vi "MultiSlit_Graphical.vi"() -> (0 "Offsets and Rotation":T7 {"Delta Y" format="%#_4g"; "Delta X" format="%#_4g"; "Delta Theta" format="%#_4g"})   [LabVIEW 2015]
doc: "A graphical tool to provide rotation and offsets needed to align a slit mask with the corresponding field on the sky, using fits images of the mask and field. Based on Brad Barlow's QuickLook software for the Goodman Spectrograph."
uses:
  gfitsio/gfitsio-refnum.ctl
  SystemUtil/Command.ctl
  SIcamera_Globals.vi
  Instance           7 27Saved   MultiSlit_Graphical .vi
  Instance           8 27Saved   MultiSlit_Graphical .vi
panel:
  out "Gauss Fit Window 2":i16[][](array[numeric])
  in  "Zoom Window Width (1/x) 2":u32=10
  out "Display Binning 2":i16
  out "Raw Image Buffer 2":i16[][](array[numeric])
  out "Display Binning":i16
  in  "# of pix to display":i32=200000
  out "Minimum Pix Value":dbl
  out "Maximum Pix Value":dbl
  out "Avg Pix Value":dbl format="%#.1f"
  out "Path to Current File":path
  out "Gauss Fit Window":i16[][](array[numeric])
  in  "Zoom Window Width (1/x)":u32=10
  out "Spectrum Status":string
  out "Image Buffer Info.":T1
  out "error IO":errorcluster
  in  "# of rows at a time":dbl=1.0
  out "Raw Image Buffer 1":i16[][](array[numeric])
  out "Raw Data":T2
  out "gfits refnum":T3
  in  "Tab Control":T4(tab)
  in  "Image Open 2":bool
  out "String 5":string="Center cursor in window - c\nCenter cursor on star or box in zoom window - r\nCenter cursor on slit - a"
  in  "LoadStar":bool
  in  "StarSelection":u16(ring) items=["Star 1", "Star 2", "Star 3"]
  out "String 2":string="Load current coordinates as "
  in  "Autoscale":bool
  in  "Redraw":bool
  in  "Zoom Out":bool
  in  "Zoom In":bool
  out "Y":dbl format="%5.1f"
  out "X":dbl format="%5.1f"
  out "Value":dbl
  out "Zoom Window":i16[][](graph) caption="0051.NGC2808_300line.fits"
  out "Status 1":string
  in  "Image Scale Stretch":cluster{dbl, dbl}(slide)={41.0, 61.0} scale=0.0..100.0
  in  "Image1":dbl[][](graph)=[[0.0]] caption="0008_Fe_ZZCeti_930_blue_long.fits"
  out "String 4":string="Center cursor in window - c\nCenter cursor on star or box in zoom window - r\nCenter cursor on slit - a"
  in  "Image Open":bool
  in  "Image Scale Stretch 2":cluster{dbl, dbl}(slide)={41.0, 61.0} scale=0.0..100.0
  in  "LoadSlit":bool
  in  "SlitSelection":u16(ring) items=["Slit 1", "Slit 2", "Slit 3"]
  out "Test":string="Load current coordinates as "
  in  "Autoscale 2":bool
  in  "Redraw 2":bool
  in  "Zoom Out 2":bool
  in  "Zoom In 2":bool
  out "Y 2":dbl format="%5.1f"
  out "X 2":dbl format="%5.1f"
  out "Value 2":dbl
  out "Zoom Window 2":i16[][](graph) caption="0051.NGC2808_300line.fits"
  out "Status 2":string
  in  "Image2":dbl[][](graph) caption="0267.WASP17b_2100_NaD.fits"
  in  "Set Values to Zero":bool
  out "new y1":dbl
  out "new x1":dbl
  out "String 3":string
  in  "Slit Positions":T5
  in  "Star Positions":T6
  in  "Send Target Offset Position":bool
  in  "Calculate Shifts":bool
  out "FITS Header 2":string
  out "FITS Header":string
  in  "CommandQ":string="MULTISLIT_Q"
  # "X Position"
  # "Y Position"
  # "Star 1"
  # "Star 2"
  # "Star 3"
  # "Slit 1"
  # "Slit 2"
  # "Slit 3"
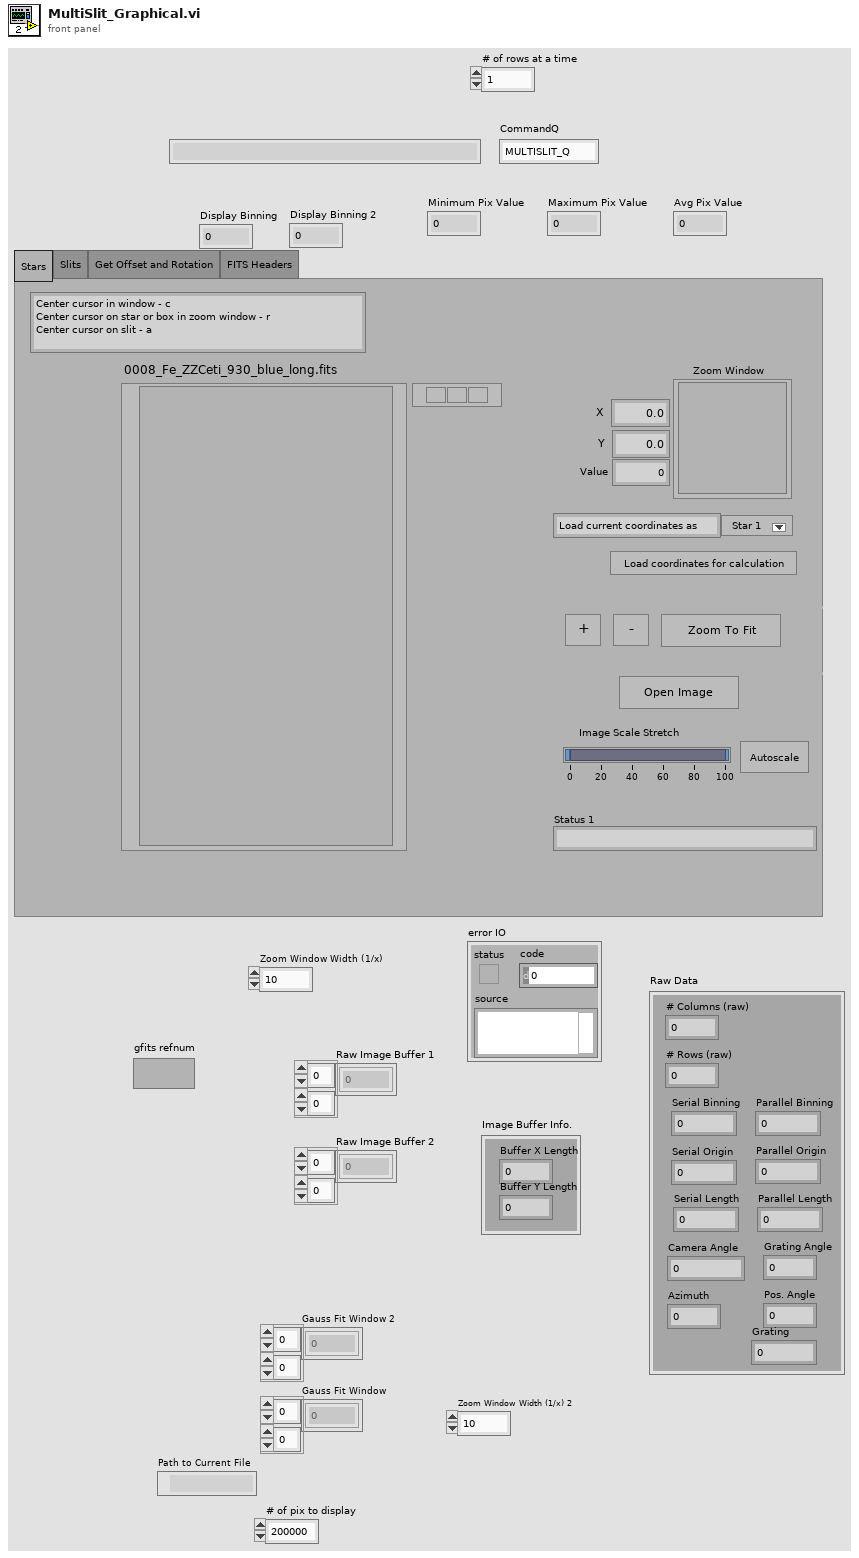
[diagram p1: front panel]
types:
  T1 = cluster{"Buffer X Length":dbl, "Buffer Y Length ":dbl}
  T2 = cluster{"# Columns (raw) ":dbl, "# Rows (raw)":dbl, "Serial Origin":dbl, "Parallel Origin":dbl, "Camera Angle":dbl, "Grating Angle":dbl, "Serial Binning":dbl, "Parallel Binning":dbl, "Azimuth":dbl, "Serial Length":dbl, "Parallel Length":dbl, "Pos. Angle":dbl, "Grating":dbl}
  T3 = typedef "gfitsio-refnum.ctl" = refnum<k1>
  T4 = enum32{"Stars", "Slits", "Get Offset and Rotation", "FITS Headers"}
  T5 = cluster{"Slit x1":dbl, "Slit x2":dbl, "Slit x3":dbl, "Slit y2":dbl, "Slit y3":dbl, "Slit y1":dbl}
  T6 = cluster{"Star x1":dbl, "Star x2":dbl, "Star x3":dbl, "Star y2":dbl, "Star y3":dbl, "Star y1":dbl}
  T7 = cluster{"Delta Theta":dbl, "Delta X":dbl, "Delta Y":dbl}
  T8 = typedef "Command.ctl" = cluster{"Command":string, "Parameter":string}
  T9 = enum32{"existing file", "new file", "new or existing file", "existing dir", "new dir", "new or existing dir", "existing file (use LLBs)", "new file (use LLBs)", "new or existing file (use LLBs)", "new or existing file or directory (use LLBs)"}
  T10 = typedef "LVRangeTypeDef.ctl" = cluster{"Minimum":dbl, "Maximum":dbl, "Increment":dbl, "Minor Increment":dbl, "Start":dbl}
  T11 = typedef "LVPoint32TypeDef.ctl" = cluster{"Horizontal":i32, "Vertical":i32}
  T12 = cluster{"Delta Theta":dbl, "Delta X":dbl, "Delta Y":dbl, "Delta Theta":dbl, "Delta X":dbl, "Delta Y":dbl}
  T13 = typedef "LVPointDoubleTypeDef.ctl" = cluster{"Cursor X":dbl, "Cursor Y":dbl}
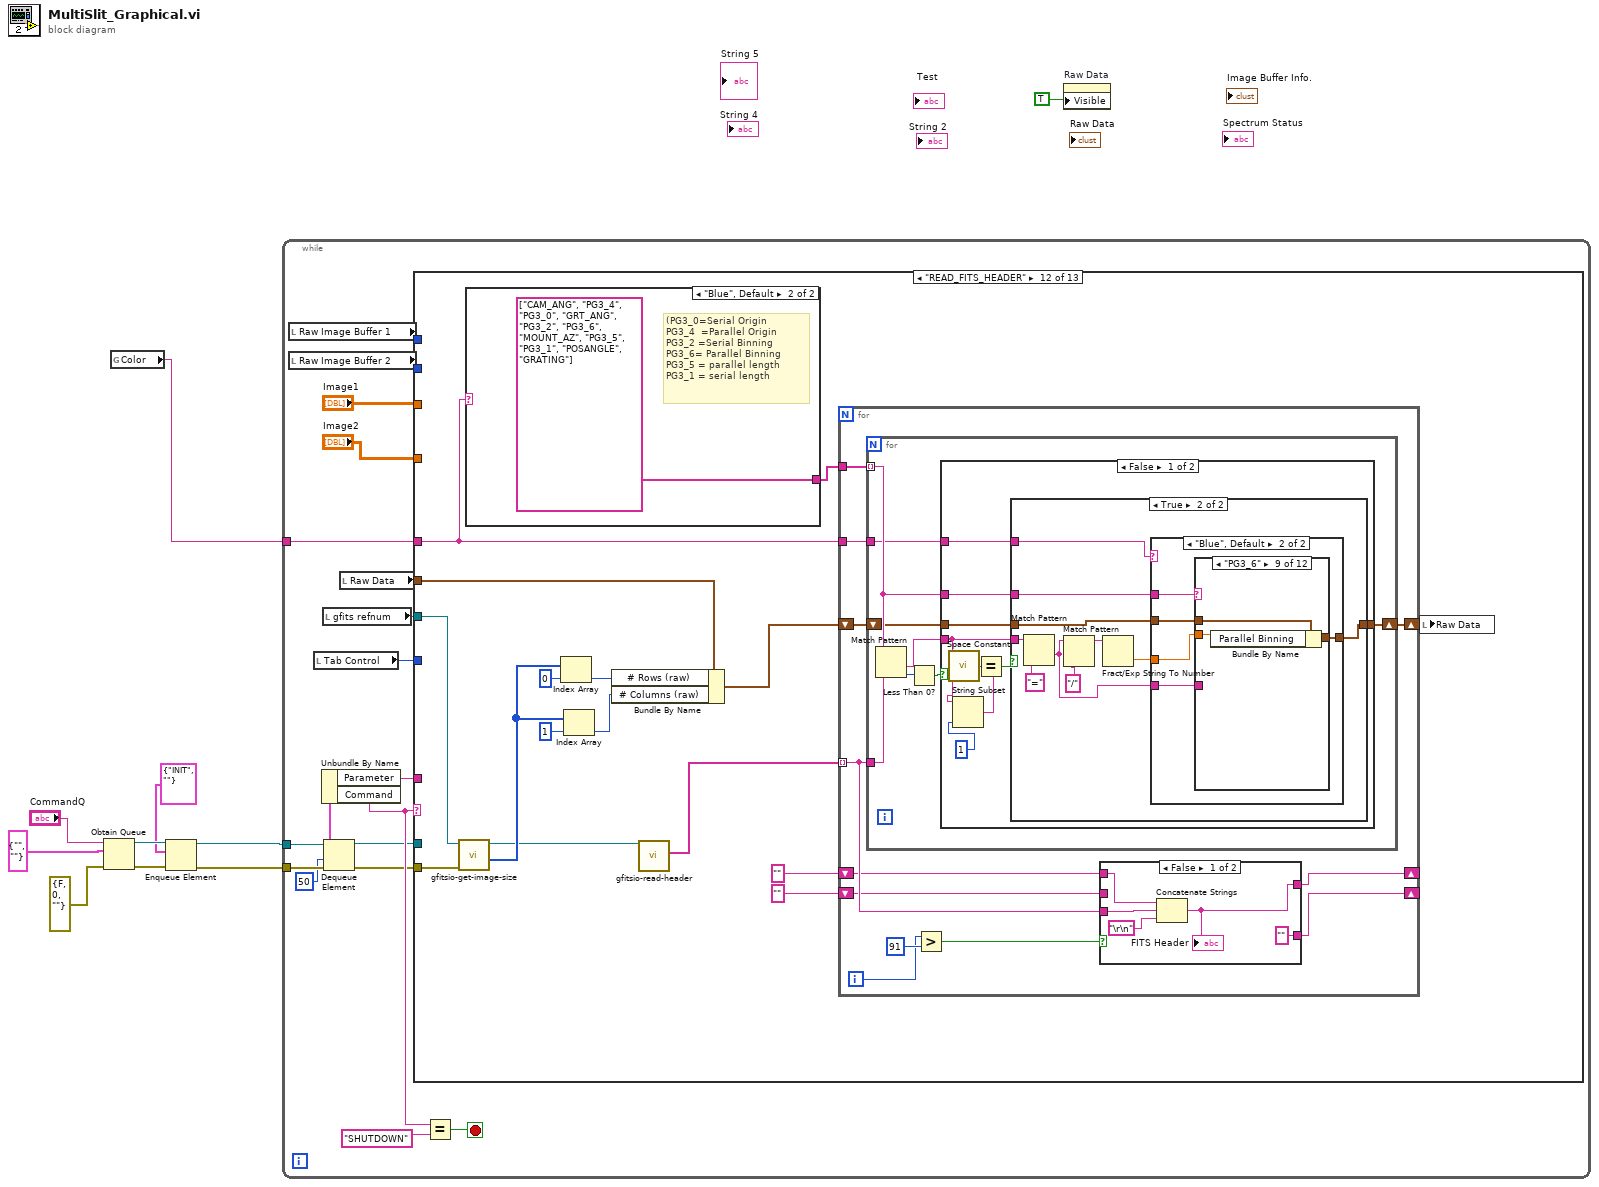
[diagram p0: block diagram]
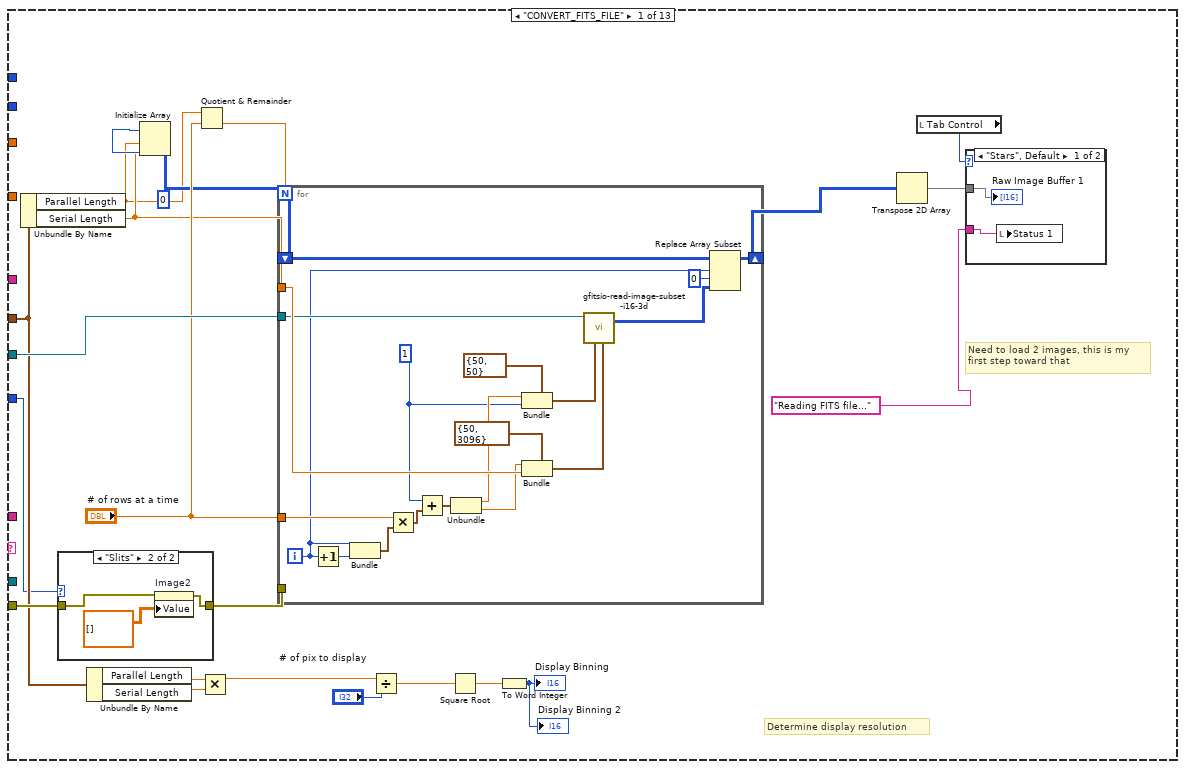
[diagram p2: hidden frame]
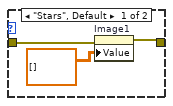
[diagram p3: hidden frame]
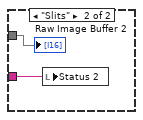
[diagram p4: hidden frame]
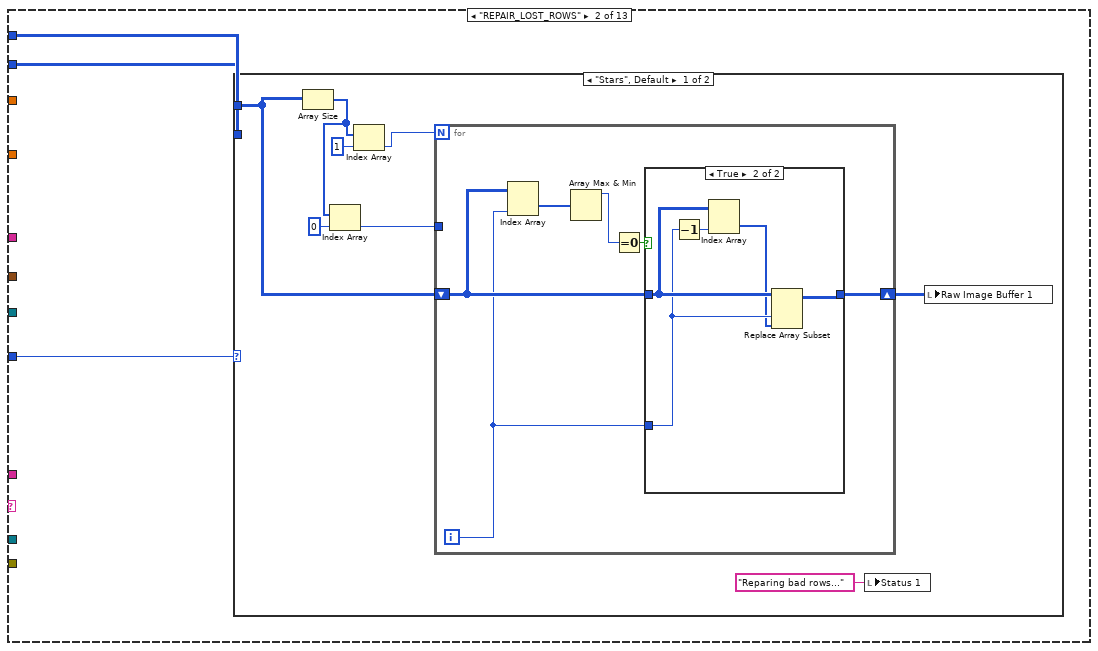
[diagram p5: hidden frame]
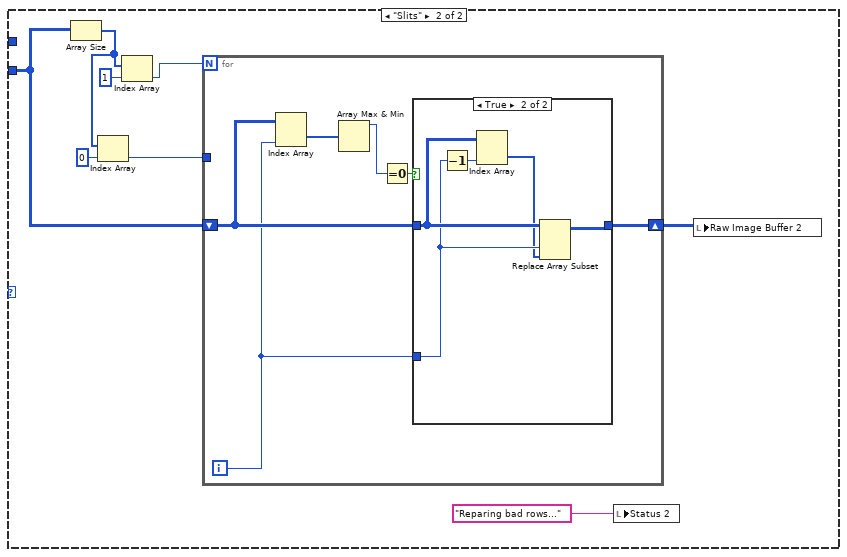
[diagram p7: hidden frame]
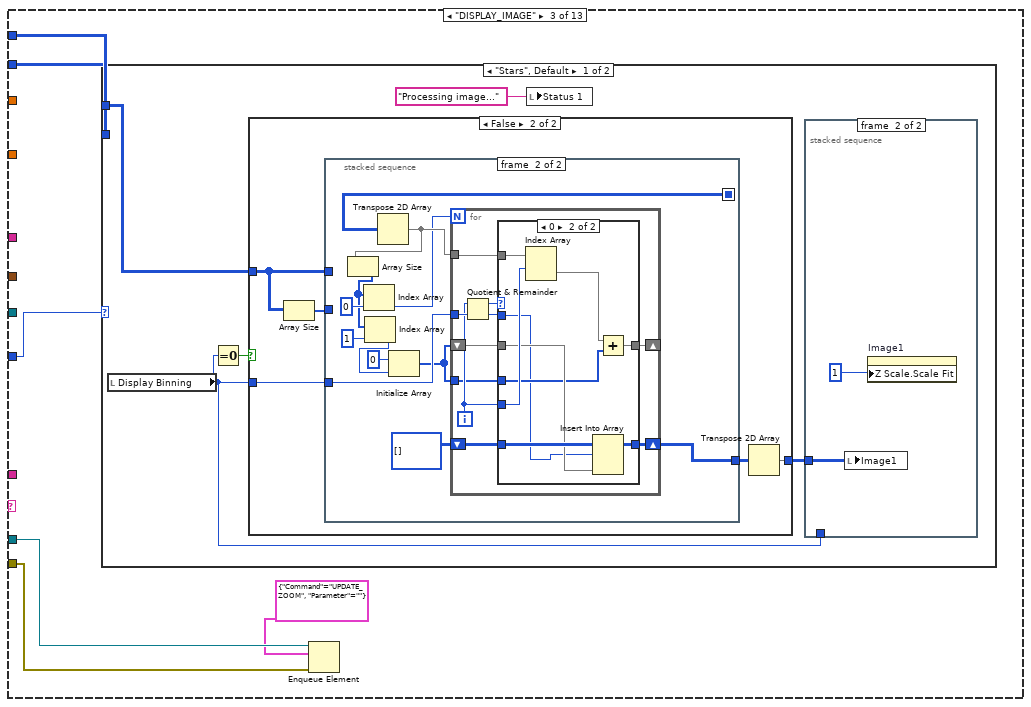
[diagram p9: hidden frame]
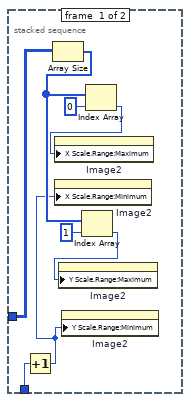
[diagram p10: hidden frame]
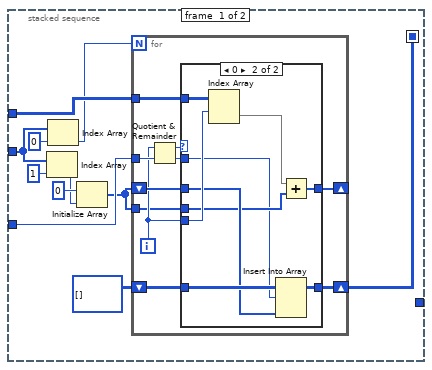
[diagram p12: hidden frame]
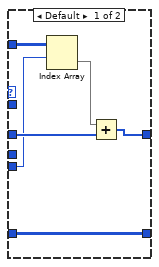
[diagram p13: hidden frame]
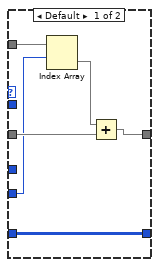
[diagram p14: hidden frame]
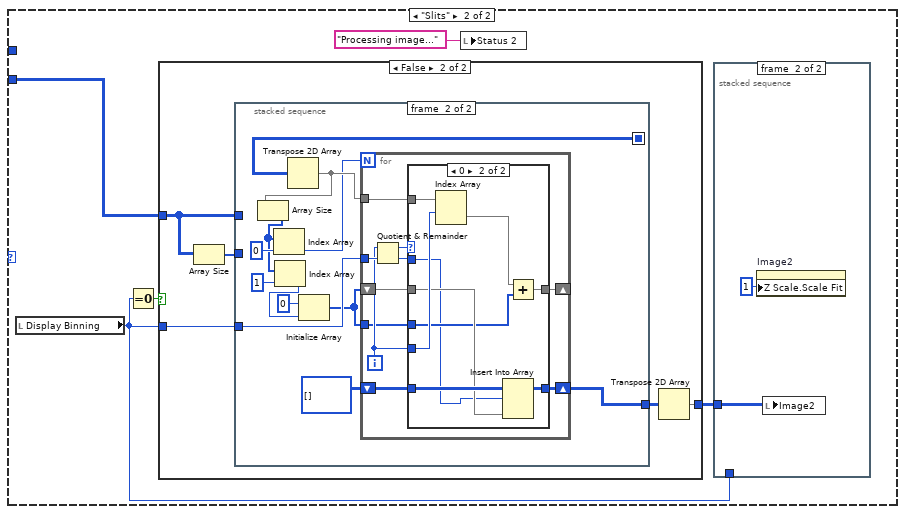
[diagram p15: hidden frame]
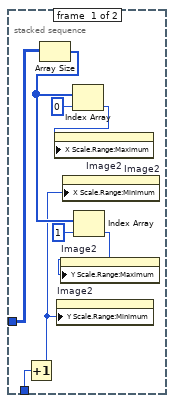
[diagram p16: hidden frame]
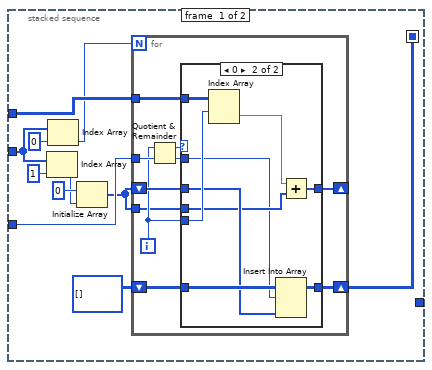
[diagram p18: hidden frame]
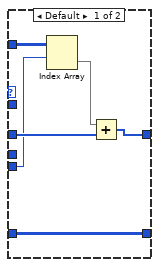
[diagram p19: hidden frame]
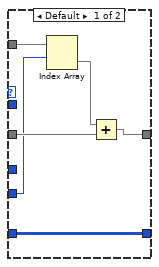
[diagram p20: hidden frame]
diagram:
  n1 = Obtain Queue(name (unnamed)="CommandQ", element data type=T8 {"Command"="", "Parameter"=""} ("Command"), error in (no error)=errorcluster {"status"=FALSE, "code"=0, "source"=""}) -> (queue out=w8:refnum<queue>, error out=w7:errorcluster)  [unwired: 2 in, 1 out]
  n2 = global read "SIcamera_Globals.vi" "Color"() -> (w1:string)
  n3 = Enqueue Element(queue=w8, element=T8 {"Command"="INIT", "Parameter"=""}, error in (no error)=w7) -> (queue out=w5:refnum<queue>, error out=w4:errorcluster)  [unwired: 1 in, 1 out]
  n4 = while {
    tunnel: w4 -> [w28]
    tunnel: w5 -> [w27]
    tunnel: w1 -> [w11]
    stop <- w24 stop-if-true
    n5 = local read "Raw Image Buffer 1"() -> (w15:i16[][])
    n6 = local read "Raw Image Buffer 2"() -> (w14:i16[][])
    n7 = local read "Tab Control"() -> (w13:T4)
    n8 = local read "gfits refnum"() -> (w18:T3)
    n9 = Dequeue Element(queue=w27, timeout in ms (-1)=50, error in (no error)=w28) -> (queue out=w21:refnum<queue>, element=w26:T8, error out=w22:errorcluster)  [unwired: 1 out]
    n10 = Unbundle By Name(w26) -> ("Parameter"=w19:string, "Command"=w23:string)
    n11 = local read "Raw Data"() -> (w17:T2)
    n12 = case shown="\"READ_FITS_HEADER\"" w23 {
      tunnel: w22 -> [w45 _ w125 _ w325 w1011 w1017 _ _ _ w1282 w1325 _]
      tunnel: w21 -> [_ _ w127 _ w326 w1012 w1018 _ _ _ w1281 _ _]
      tunnel: w19 -> [_ _ _ _ _ _ _ _ _ _ w1274 _ _]
      tunnel: "Image1" -> [_ _ _ _ w324 _ _ _ _ _ _ _ _]
      tunnel: w18 -> [w50 _ _ _ _ _ _ _ _ _ _ w1326 _]
      tunnel: w17 -> [w41 _ _ _ w323 _ w1016 _ _ _ _ w1323 _]
      tunnel: w15 -> [_ w82 w128 _ w322 _ _ _ w1147 w1212 _ _ w1474]
      tunnel: w14 -> [_ w81 w123 _ w319 _ _ _ w1146 w1211 _ _ w1473]
      tunnel: w13 -> [w31 w80 w124 _ w320 _ w1013 w1113 w1148 w1213 w1271 _ w1475]
      tunnel: "Image2" -> [_ _ _ _ w321 _ _ _ _ _ _ _ _]
      tunnel: w11 -> [_ _ _ _ _ _ _ _ _ _ _ w1316 _]
      frame "CONVERT_FITS_FILE" {
        # "Need to load 2 images, this is my\nfirst step toward that"
        # "Determine display resolution"
        n13 = Unbundle By Name(w41) -> ("Parallel Length"=w34:dbl, "Serial Length"=w42:dbl)
        n14 = case shown="\"Slits\"" w31 {
          tunnel: [w53 w56] -> w46
          tunnel: w45 -> [w52 w55]
          frame "Stars", Default {
            n15 = property on="Image1" class="IntGraph (strict)"(error in=w52, "Value"=dbl[][] [] ("Image")) -> (error out=w53:errorcluster)  [unwired: 1 in, 1 out]
          }
          frame "Slits" {
            n16 = property on="Image2" class="IntGraph (strict)"(error in=w55, "Value"=dbl[][] [] ("Image")) -> (error out=w56:errorcluster)  [unwired: 1 in, 1 out]
          }
        }
        n17 = Unbundle By Name(w41) -> ("Parallel Length"=w40:dbl, "Serial Length"=w39:dbl)
        n18 = Initialize Array(i16 0 ("element"), w34, w42) -> (w44:i16[][])
        n19 = Quotient & Remainder(x=w34, y="# of rows at a time") -> (floor(x/y)=w49:dbl)  [unwired: 1 out]
        n20 = Multiply(x=w40, y=w39) -> (x*y=w37:dbl)
        n21 = for {
          N: w49 -> [_]
          tunnel: w42 -> [w78]
          tunnel: w50 -> [w68]
          tunnel: "# of rows at a time" -> [w77]
          shift-right: [w65] -> w47
          shift-left: w44 -> [w64]
          tunnel: w46 -> [_]
          i -> [w63]
          w70 = 1
          n22 = Increment(x=w63) -> (x+1=w74:i32)
          n23 = Bundle(w63, w74) -> (w75:cluster{i32, i32})  [unwired: 1 in]
          n24 = Multiply(x=w77, y=w75) -> (x*y=w76:cluster{dbl, dbl})
          n25 = Add(x=w70, y=w76) -> (x+y=w73:cluster{dbl, dbl})
          n26 = Unbundle(w73) -> (w71:dbl, w72:dbl)
          n27 = Bundle(cluster=cluster{i32, i32} {50, 50} ("fpixel (1,1,1)"), w71, w70) -> (w67:cluster{i32, i32})
          n28 = Bundle(cluster=cluster{i32, i32} {50, 3096} ("lpixel (-1,-1,-1: rest)"), w72, w78) -> (w66:cluster{i32, i32})
          n29 = call "gfitsio-read-image-subset-i16-3d.vi"("lpixel (-1,-1,-1: rest)"=w66, "fpixel (1,1,1)"=w67, "gfits refnum"=w68) -> ("data"=w61:i16[][])  [unwired: 5 in, 3 out]
          n30 = Replace Array Subset(array=w64, new element=w61, index (row)=w63, index (col)=0 ("disabled index (col)")) -> (w65:i16[][])
        }
        n31 = Divide(x=w37, y="# of pix to display") -> (x/y=w36:dbl)
        n32 = Square Root(x=w36) -> (sqrt(x)=w35:dbl)
        n33 = To Word Integer(number=w35) -> (16bit integer=→"Display Binning" →"Display Binning 2":i16)
        n34 = Transpose 2D Array(2D array=w47) -> (transposed array=w32:i16[][])
        n35 = local read "Tab Control"() -> (w33:T4)
        n36 = case shown="\"Stars\", Default" w33 {
          tunnel: w32 -> [w58 w60]
          tunnel: "Reading FITS file..." ("Status") -> [w57 w59]
          frame "Stars", Default {
            n37 = local write "Status 1"(w57) -> ()
            "Raw Image Buffer 1" <- w58
          }
          frame "Slits" {
            n38 = local write "Status 2"(w59) -> ()
            "Raw Image Buffer 2" <- w60
          }
        }
      }
      frame "REPAIR_LOST_ROWS" {
        n39 = case shown="\"Stars\", Default" w80 {
          tunnel: w82 -> [w85 _]
          tunnel: w81 -> [_ w105]
          frame "Stars", Default {
            n40 = Array Size(array=w85) -> (size(s)=w87:i32[])
            n41 = Index Array(array=w87, index=0) -> (element=w86:i32)
            n42 = Index Array(array=w87, index=1) -> (element=w89:i32)
            n43 = for {
              N: w89 -> [_]
              shift-right: [w96] -> w84
              shift-left: w85 -> [w95]
              tunnel: w86 -> [_]
              i -> [w94]
              n44 = Index Array(array=w95, index (col)=w94) -> (element=w93:i16[])  [unwired: 1 in]
              n45 = Array Max & Min(array=w93) -> (max value=w91:i16)  [unwired: 3 out]
              n46 = Equal To 0?(x=w91) -> (x = 0?=w92:bool)
              n47 = case shown="True" w92 {
                tunnel: w94 -> [_ w99]
                tunnel: w95 -> [w97 w101]
                tunnel: [w97 w102] -> w96
                frame False {
                }
                frame True {
                  n48 = Decrement(x=w99) -> (x-1=w100:i32)
                  n49 = Index Array(array=w101, index (col)=w100) -> (element=w98:i16[])  [unwired: 1 in]
                  n50 = Replace Array Subset(array=w101, new element=w98, index (col)=w99) -> (w102:i16[][])  [unwired: 1 in]
                }
              }
            }
            n51 = local write "Status 1"("Reparing bad rows..." ("Image Status")) -> ()
            n52 = local write "Raw Image Buffer 1"(w84) -> ()
          }
          frame "Slits" {
            n53 = Array Size(array=w105) -> (size(s)=w107:i32[])
            n54 = Index Array(array=w107, index=0) -> (element=w106:i32)
            n55 = Index Array(array=w107, index=1) -> (element=w109:i32)
            n56 = for {
              N: w109 -> [_]
              shift-right: [w116] -> w104
              shift-left: w105 -> [w115]
              tunnel: w106 -> [_]
              i -> [w114]
              n57 = Index Array(array=w115, index (col)=w114) -> (element=w113:i16[])  [unwired: 1 in]
              n58 = Array Max & Min(array=w113) -> (max value=w111:i16)  [unwired: 3 out]
              n59 = Equal To 0?(x=w111) -> (x = 0?=w112:bool)
              n60 = case shown="True" w112 {
                tunnel: w114 -> [_ w119]
                tunnel: w115 -> [w117 w121]
                tunnel: [w117 w122] -> w116
                frame False {
                }
                frame True {
                  n61 = Decrement(x=w119) -> (x-1=w120:i32)
                  n62 = Index Array(array=w121, index (col)=w120) -> (element=w118:i16[])  [unwired: 1 in]
                  n63 = Replace Array Subset(array=w121, new element=w118, index (col)=w119) -> (w122:i16[][])  [unwired: 1 in]
                }
              }
            }
            n64 = local write "Status 2"("Reparing bad rows..." ("Image Status")) -> ()
            n65 = local write "Raw Image Buffer 2"(w104) -> ()
          }
        }
      }
      frame "DISPLAY_IMAGE" {
        n66 = case shown="\"Stars\", Default" w124 {
          tunnel: w128 -> [w132 _]
          tunnel: w123 -> [_ w223]
          frame "Stars", Default {
            n67 = local read "Display Binning"() -> (w130:i16)
            n68 = Equal To 0?(x=w130) -> (x = 0?=w131:bool)
            n69 = case shown="False" w131 {
              tunnel: w132 -> [w144 w148]
              tunnel: w130 -> [_ w147]
              tunnel: [w144 w146] -> w129
              frame True {
              }
              frame False {
                n70 = Array Size(array=w148) -> (size(s)=w149:i32[])
                n71 = stacked-sequence {
                  seq-local: [w158 _] -> [_ w195]
                  tunnel: w148 -> [w160 _]
                  tunnel: w149 -> [w152 _]
                  tunnel: w147 -> [w156 w192]
                  tunnel: [_ w196] -> w145
                  frame #0 {
                    n72 = Index Array(array=w152, index=1) -> (element=w151:i32)
                    n73 = Index Array(array=w152, index=0) -> (element=w154:i32)
                    n74 = Initialize Array(0 ("element"), w151) -> (w150:i32[])
                    n75 = for {
                      N: w154 -> [_]
                      tunnel: w160 -> [w170]
                      shift-right: [w168] -> w158
                      shift-left: i32[][] [] -> [w169]
                      tunnel: w156 -> [w167]
                      shift-right: [w163] -> _
                      shift-left: w150 -> [w164]
                      tunnel: w150 -> [w161]
                      i -> [w162]
                      n76 = Quotient & Remainder(x=w162, y=w167) -> (x-y*floor(x/y)=w166:i32, floor(x/y)=w165:i32)
                      n77 = case shown="0" w166 {
                        tunnel: w170 -> [w176 w185]
                        tunnel: w162 -> [w172 w182]
                        tunnel: w169 -> [w171 w184]
                        tunnel: [w171 w183] -> w168
                        tunnel: w165 -> [_ w177]
                        tunnel: w164 -> [w174 w181]
                        tunnel: [w173 w179] -> w163
                        tunnel: w161 -> [_ w178]
                        frame Default {
                          n78 = Index Array(array=w176, index (row)=w172) -> (element=w175:i16[])  [unwired: 1 in]
                          n79 = Add(x=w175, y=w174) -> (x+y=w173:i32[])
                        }
                        frame 0 {
                          n80 = Index Array(array=w185, index (row)=w182) -> (element=w180:i16[])  [unwired: 1 in]
                          n81 = Insert Into Array(array=w184, index (row)=w177, new element=w181) -> (w183:i32[][])  [unwired: 1 in]
                          n82 = Add(x=w180, y=w178) -> (x+y=w179:i32[])
                        }
                      }
                    }
                  }
                  frame #1 {
                    n83 = Transpose 2D Array(2D array=w195) -> (transposed array=w193:i32[][])
                    n84 = Array Size(array=w193) -> (size(s)=w187:i32[])
                    n85 = Index Array(array=w187, index=0) -> (element=w190:i32)
                    n86 = Index Array(array=w187, index=1) -> (element=w188:i32)
                    n87 = Initialize Array(0 ("element"), w188) -> (w186:i32[])
                    n88 = for {
                      N: w190 -> [_]
                      tunnel: w193 -> [w207]
                      shift-right: [w200] -> w196
                      shift-left: i32[][] [] -> [w201]
                      shift-right: [w206] -> _
                      shift-left: w186 -> [w205]
                      tunnel: w192 -> [w202]
                      tunnel: w186 -> [w198]
                      i -> [w199]
                      n89 = Quotient & Remainder(x=w199, y=w202) -> (x-y*floor(x/y)=w204:i32, floor(x/y)=w203:i32)
                      n90 = case shown="0" w204 {
                        tunnel: w207 -> [w213 w222]
                        tunnel: w199 -> [w209 w219]
                        tunnel: w201 -> [w208 w221]
                        tunnel: [w208 w220] -> w200
                        tunnel: w203 -> [_ w214]
                        tunnel: w205 -> [w211 w218]
                        tunnel: [w210 w216] -> w206
                        tunnel: w198 -> [_ w215]
                        frame Default {
                          n91 = Index Array(array=w213, index (row)=w209) -> (element=w212:i32[])  [unwired: 1 in]
                          n92 = Add(x=w212, y=w211) -> (x+y=w210:i32[])
                        }
                        frame 0 {
                          n93 = Index Array(array=w222, index (row)=w219) -> (element=w217:i32[])  [unwired: 1 in]
                          n94 = Insert Into Array(array=w221, index (row)=w214, new element=w218) -> (w220:i32[][])  [unwired: 1 in]
                          n95 = Add(x=w217, y=w215) -> (x+y=w216:i32[])
                        }
                      }
                    }
                  }
                }
                n96 = Transpose 2D Array(2D array=w145) -> (transposed array=w146:i32[][])
              }
            }
            n97 = local write "Status 1"("Processing image..." ("Status")) -> ()
            n98 = stacked-sequence {
              tunnel: w130 -> [w139 _]
              tunnel: w129 -> [w140 w143]
              frame #0 {
                n99 = Increment(x=w139) -> (x+1=w134:i16)
                n100 = Array Size(array=w140) -> (size(s)=w136:i32[])
                n101 = property on="Image2" class="IntGraph (strict)"("X Scale.Range:Minimum"=w134) -> ()  [unwired: 2 in, 2 out]
                n102 = property on="Image2" class="IntGraph (strict)"("Y Scale.Range:Minimum"=w134) -> ()  [unwired: 2 in, 2 out]
                n103 = Index Array(array=w136, index=1) -> (element=w135:i32)
                n104 = property on="Image2" class="IntGraph (strict)"("Y Scale.Range:Maximum"=w135) -> ()  [unwired: 2 in, 2 out]
                n105 = Index Array(array=w136, index=0) -> (element=w138:i32)
                n106 = property on="Image2" class="IntGraph (strict)"("X Scale.Range:Maximum"=w138) -> ()  [unwired: 2 in, 2 out]
              }
              frame #1 {
                n107 = local write "Image1"(w143) -> ()
                n108 = property on="Image1" class="IntGraph (strict)"("Z Scale.Scale Fit"=1) -> ()  [unwired: 2 in, 2 out]
              }
            }
          }
          frame "Slits" {
            n109 = local read "Display Binning"() -> (w224:i16)
            n110 = Equal To 0?(x=w224) -> (x = 0?=w226:bool)
            n111 = case shown="False" w226 {
              tunnel: w223 -> [w238 w242]
              tunnel: w224 -> [_ w241]
              tunnel: [w238 w240] -> w225
              frame True {
              }
              frame False {
                n112 = Array Size(array=w242) -> (size(s)=w243:i32[])
                n113 = stacked-sequence {
                  seq-local: [w252 _] -> [_ w289]
                  tunnel: w242 -> [w254 _]
                  tunnel: w243 -> [w246 _]
                  tunnel: w241 -> [w250 w286]
                  tunnel: [_ w290] -> w239
                  frame #0 {
                    n114 = Index Array(array=w246, index=1) -> (element=w245:i32)
                    n115 = Index Array(array=w246, index=0) -> (element=w248:i32)
                    n116 = Initialize Array(0 ("element"), w245) -> (w244:i32[])
                    n117 = for {
                      N: w248 -> [_]
                      tunnel: w254 -> [w264]
                      shift-right: [w262] -> w252
                      shift-left: i32[][] [] -> [w263]
                      tunnel: w250 -> [w261]
                      shift-right: [w257] -> _
                      shift-left: w244 -> [w258]
                      tunnel: w244 -> [w255]
                      i -> [w256]
                      n118 = Quotient & Remainder(x=w256, y=w261) -> (x-y*floor(x/y)=w260:i32, floor(x/y)=w259:i32)
                      n119 = case shown="0" w260 {
                        tunnel: w264 -> [w270 w279]
                        tunnel: w256 -> [w266 w276]
                        tunnel: w263 -> [w265 w278]
                        tunnel: [w265 w277] -> w262
                        tunnel: w259 -> [_ w271]
                        tunnel: w258 -> [w268 w275]
                        tunnel: [w267 w273] -> w257
                        tunnel: w255 -> [_ w272]
                        frame Default {
                          n120 = Index Array(array=w270, index (row)=w266) -> (element=w269:i16[])  [unwired: 1 in]
                          n121 = Add(x=w269, y=w268) -> (x+y=w267:i32[])
                        }
                        frame 0 {
                          n122 = Index Array(array=w279, index (row)=w276) -> (element=w274:i16[])  [unwired: 1 in]
                          n123 = Insert Into Array(array=w278, index (row)=w271, new element=w275) -> (w277:i32[][])  [unwired: 1 in]
                          n124 = Add(x=w274, y=w272) -> (x+y=w273:i32[])
                        }
                      }
                    }
                  }
                  frame #1 {
                    n125 = Transpose 2D Array(2D array=w289) -> (transposed array=w287:i32[][])
                    n126 = Array Size(array=w287) -> (size(s)=w281:i32[])
                    n127 = Index Array(array=w281, index=0) -> (element=w284:i32)
                    n128 = Index Array(array=w281, index=1) -> (element=w282:i32)
                    n129 = Initialize Array(0 ("element"), w282) -> (w280:i32[])
                    n130 = for {
                      N: w284 -> [_]
                      tunnel: w287 -> [w301]
                      shift-right: [w294] -> w290
                      shift-left: i32[][] [] -> [w295]
                      shift-right: [w300] -> _
                      shift-left: w280 -> [w299]
                      tunnel: w286 -> [w296]
                      tunnel: w280 -> [w292]
                      i -> [w293]
                      n131 = Quotient & Remainder(x=w293, y=w296) -> (x-y*floor(x/y)=w298:i32, floor(x/y)=w297:i32)
                      n132 = case shown="0" w298 {
                        tunnel: w301 -> [w307 w316]
                        tunnel: w293 -> [w303 w313]
                        tunnel: w295 -> [w302 w315]
                        tunnel: [w302 w314] -> w294
                        tunnel: w297 -> [_ w308]
                        tunnel: w299 -> [w305 w312]
                        tunnel: [w304 w310] -> w300
                        tunnel: w292 -> [_ w309]
                        frame Default {
                          n133 = Index Array(array=w307, index (row)=w303) -> (element=w306:i32[])  [unwired: 1 in]
                          n134 = Add(x=w306, y=w305) -> (x+y=w304:i32[])
                        }
                        frame 0 {
                          n135 = Index Array(array=w316, index (row)=w313) -> (element=w311:i32[])  [unwired: 1 in]
                          n136 = Insert Into Array(array=w315, index (row)=w308, new element=w312) -> (w314:i32[][])  [unwired: 1 in]
                          n137 = Add(x=w311, y=w309) -> (x+y=w310:i32[])
                        }
                      }
                    }
                  }
                }
                n138 = Transpose 2D Array(2D array=w239) -> (transposed array=w240:i32[][])
              }
            }
            n139 = local write "Status 2"("Processing image..." ("Status")) -> ()
            n140 = stacked-sequence {
              tunnel: w225 -> [w230 w237]
              tunnel: w224 -> [w229 _]
              frame #0 {
                n141 = Increment(x=w229) -> (x+1=w228:i16)
                n142 = Array Size(array=w230) -> (size(s)=w233:i32[])
                n143 = property on="Image2" class="IntGraph (strict)"("Y Scale.Range:Minimum"=w228) -> ()  [unwired: 2 in, 2 out]
                n144 = property on="Image2" class="IntGraph (strict)"("X Scale.Range:Minimum"=w228) -> ()  [unwired: 2 in, 2 out]
                n145 = Index Array(array=w233, index=0) -> (element=w234:i32)
                n146 = property on="Image2" class="IntGraph (strict)"("X Scale.Range:Maximum"=w234) -> ()  [unwired: 2 in, 2 out]
                n147 = Index Array(array=w233, index=1) -> (element=w231:i32)
                n148 = property on="Image2" class="IntGraph (strict)"("Y Scale.Range:Maximum"=w231) -> ()  [unwired: 2 in, 2 out]
              }
              frame #1 {
                n149 = property on="Image2" class="IntGraph (strict)"("Z Scale.Scale Fit"=u8 1) -> ()  [unwired: 2 in, 2 out]
                n150 = local write "Image2"(w237) -> ()
              }
            }
          }
        }
        n151 = Enqueue Element(queue=w127, element=T8 {"Command"="UPDATE_ZOOM", "Parameter"=""}, error in (no error)=w125) -> ()  [unwired: 1 in, 3 out]
      }
      frame "INIT" {
        w317 = dbl[][] [[0.0]] ("Image")
        w318 = dbl[][] [[0.0]] ("Image")
        n152 = local write "Zoom Window"(w318) -> ()
        n153 = local write "Image1"(w318) -> ()
        n154 = local write "Zoom Window 2"(w317) -> ()
        n155 = local write "Image2"(w317) -> ()
      }
      frame "", Default {
        n156 = event shown="[2] Menu Selection (User)" {
          selector: _ -> [_ _ _ _ _ _ _ _ _ _ _ _ _ _ _ _ _ _ _ _ _ _ _]
          dyn-events: _ -> [_ _ _ _ _ _ _ _ _ _ _ _ _ _ _ _ _ _ _ _ _ _ _]
          timeout: 50 -> [_ _ _ _ _ _ _ _ _ _ _ _ _ _ _ _ _ _ _ _ _ _ _]
          tunnel: w326 -> [_ w342 w349 _ _ w411 w415 w431 w445 w451 _ _ _ _ _ w884 w914 _ _ w976 w979 _ _]
          tunnel: w325 -> [_ w343 w348 _ _ w412 w414 w430 w444 w452 _ _ _ _ _ w885 w913 _ _ w975 w978 _ _]
          tunnel: w324 -> [_ _ _ _ _ _ _ _ _ w448 _ _ _ _ _ w886 _ _ _ _ _ _ _]
          tunnel: w323 -> [_ _ _ _ _ _ _ _ _ w450 _ _ _ _ _ _ _ _ _ _ _ _ _]
          tunnel: w322 -> [_ w341 _ _ _ _ _ _ _ _ _ _ _ _ _ _ _ _ _ _ _ _ _]
          tunnel: w321 -> [_ _ _ _ _ _ _ _ _ w447 _ _ _ _ _ _ _ _ _ _ _ _ _]
          tunnel: w320 -> [_ _ _ _ _ _ _ _ _ w453 _ _ _ _ _ _ _ _ _ _ _ _ _]
          tunnel: w319 -> [_ w340 _ _ _ _ _ _ _ _ _ _ _ _ _ _ _ _ _ _ _ _ _]
          event Timeout {
            n157 = event-data() -> ()  [unwired: 1 in, 2 out]
            n158 = local read "Status 2"() -> (w329:string)
            n159 = local read "Status 1"() -> (w331:string)
            n160 = case shown="Default" w331 {
              selector: w331 -> [w336 _ _ _]
              tunnel: [w336 "DONE:  Image updated" ("Image Status") "DONE:  Image re-scaled" ("Image Status") "DONE:  Star centered" ("Image Status")] -> w330
              frame Default {
              }
              frame "Processing image..." {
              }
              frame "Scaling image..." {
              }
              frame "Centering star..." {
              }
            }
            "Status 1" <- w330
            n161 = case shown="Default" w329 {
              selector: w329 -> [w332 _ _ _]
              tunnel: [w332 "DONE:  Image updated" ("Image Status") "DONE:  Image re-scaled" ("Image Status") "DONE:  Star centered" ("Image Status")] -> w328
              frame Default {
              }
              frame "Processing image..." {
              }
              frame "Scaling image..." {
              }
              frame "Centering star..." {
              }
            }
            "Status 2" <- w328
          }
          event "Tab Control": Value Change {
            n162 = event-data() -> ("NewVal"=w344:T4)  [unwired: 1 in]
            n163 = case shown="\"Get Offset and Rotation\"" w344 {
              tunnel: w341 -> [_ _ _ _]
              tunnel: w343 -> [_ _ _ w346]
              tunnel: w342 -> [_ _ _ w345]
              tunnel: w340 -> [_ _ _ _]
              frame "Stars", Default {
              }
              frame "Slits" {
              }
              frame "Get Offset and Rotation" {
              }
              frame "FITS Headers" {
                n164 = Enqueue Element(queue=w345, element=T8 {"Command"="GET_IMAGE_STATS", "Parameter"=""}, error in (no error)=w346) -> ()  [unwired: 1 in, 3 out]
              }
            }
          }
          event Menu Selection (User) {
            n165 = event-data() -> ("ItemTag"=w350:string)  [unwired: 1 in]
            n166 = case shown="\"COPY_OTHER\"" w350 {
              tunnel: w349 -> [_ w353 _ _ w393 _ _]
              tunnel: w348 -> [_ w352 _ _ w394 _ _]
              frame "", Default {
              }
              frame "EXIT" {
                n167 = Enqueue Element(queue=w353, element=T8 {"Command"="SHUTDOWN", "Parameter"=""}, error in (no error)=w352) -> ()  [unwired: 1 in, 3 out]
              }
              frame "COPY_CURRENT" {
                w359 = " " ("string")
                n168 = local read "Path to Current File"() -> (w365:path)
                n169 = Strip Path(path=w365) -> (name=w364:string)  [unwired: 1 out]
                n170 = Path To String(path=w365) -> (string=w360:string)
                n171 = Concatenate Strings("\\\\soaric7.ctio.noao.edu\\ic7home3\\observer\\today\\" ("string"), w364) -> (w358:string)
                n172 = Concatenate Strings("cmd /C" ("string"), w359, "copy" ("string"), w359, w360, w359, w358) -> (w357:string)
                n173 = call <vilib>:"System Exec.vi"("run minimized? (F)"=TRUE, "wait until completion? (T)"=TRUE, "command line"=w357) -> ("standard output"=w354:string)  [unwired: 5 in, 3 out]
                n174 = local write "Status 1"(w354) -> ()
              }
              frame "COPY_OTHER" {
                (unwired) T9."existing file" ("select mode (2)")
                n175 = File Dialog(5:"Copy to IC7" ("button label"), 6:"*.fits" ("default name"), 7:"Select an Image to Copy to Soaric7" ("prompt"), 11:path "C:/DATA" ("start path")) -> (0:w366:errorcluster, 1:w368:bool, 3:w369:path)  [unwired: 3 in, 1 out]
                n176 = Unbundle(w366) -> ()  [unwired: 3 out]
                n177 = case shown="False" w368 {
                  tunnel: w369 -> [_ w374]
                  frame True {
                  }
                  frame False {
                    w380 = " " ("string")
                    n178 = Strip Path(path=w374) -> (name=w384:string)  [unwired: 1 out]
                    n179 = Path To String(path=w374) -> (string=w381:string)
                    n180 = Concatenate Strings("\\\\soaric7.ctio.noao.edu\\ic7home3\\observer\\today\\" ("string"), w384) -> (w379:string)
                    n181 = Concatenate Strings("cmd /C" ("string"), w380, "copy" ("string"), w380, w381, w380, w379) -> (w378:string)
                    n182 = call <vilib>:"System Exec.vi"("run minimized? (F)"=TRUE, "wait until completion? (T)"=TRUE, "command line"=w378) -> ("standard output"=w373:string)  [unwired: 5 in, 3 out]
                    n183 = local write "Status 1"(w373) -> ()
                  }
                }
              }
              frame "OPEN" {
                (unwired) T9."existing file" ("select mode (2)")
                n184 = File Dialog(5:"Open Image" ("button label"), 6:"*.fits" ("default name"), 7:"Open Image" ("prompt"), 11:path "C:/DATA" ("start path")) -> (0:w385:errorcluster, 1:w392:bool, 3:w386:path)  [unwired: 3 in, 1 out]
                n185 = Unbundle(w385) -> ()  [unwired: 3 out]
                n186 = Path To String(path=w386) -> (string=w387:string)
                n187 = case shown="False" w392 {
                  tunnel: w394 -> [_ w400]
                  tunnel: w393 -> [_ w399]
                  tunnel: w387 -> [_ w397]
                  frame True {
                  }
                  frame False {
                    n188 = Bundle By Name(cluster=T8 {"Command"="", "Parameter"=""} ("element"), "Command"="OPEN_FITS_FILE", "Parameter"=w397) -> (w398:T8)
                    n189 = Enqueue Element(queue=w399, element=w398, error in (no error)=w400) -> ()  [unwired: 1 in, 3 out]
                  }
                }
              }
              frame "CONFIG" {
                n190 = call "Configuration Parameters"() -> ("# of pixels to display"=w401:dbl, "OK"=w402:bool)  [unwired: 17 in, 1 out]
                n191 = case shown="True" w402 {
                  tunnel: w401 -> [_ w404]
                  frame False {
                  }
                  frame True {
                    w405 = 40000.0 ("y")
                    n192 = Less?(x=w404, y=w405) -> (x < y?=w406:bool)
                    n193 = Select(t=w405, s=w406, f=w404) -> (s? t:f=w403:dbl)
                    n194 = local write "# of pix to display"(w403) -> ()
                  }
                }
              }
              frame "QUICK_HELP" {
                n195 = call "Display Message to User"() -> ()  [unwired: 10 in, 2 out]
              }
            }
          }
          event "Autoscale": Value Change {
            n196 = event-data() -> ()  [unwired: 1 in, 6 out]
            n197 = property on="Image1" class="IntGraph (strict)"("Z Scale.Scale Fit"=u8 1) -> ()  [unwired: 2 in, 2 out]
            n198 = local write "Autoscale"(FALSE ("Autoscale")) -> ()
          }
          event "Autoscale 2": Value Change {
            n199 = event-data() -> ()  [unwired: 1 in, 6 out]
            n200 = property on="Image2" class="IntGraph (strict)"("Z Scale.Scale Fit"=u8 1) -> ()  [unwired: 2 in, 2 out]
            n201 = local write "Autoscale 2"(FALSE ("Autoscale")) -> ()
          }
          event "Redraw": Mouse Down {
            n202 = event-data() -> ()  [unwired: 1 in, 8 out]
            n203 = Enqueue Element(queue=w411, element=T8 {"Command"="DISPLAY_IMAGE", "Parameter"=""}, error in (no error)=w412) -> ()  [unwired: 1 in, 3 out]
          }
          event "Image Open": Mouse Down {
            n204 = event-data() -> ()  [unwired: 1 in, 8 out]
            n205 = case shown="True" "Image Open" {
              tunnel: w414 -> [w421 _]
              tunnel: w415 -> [w420 _]
              frame True {
                (unwired) T9."existing file" ("select mode (2)")
                n206 = File Dialog(5:"Open Image" ("button label"), 6:"*.fits" ("default name"), 7:"Open Image" ("prompt"), 11:path "C:/DATA" ("start path")) -> (0:w417:errorcluster, 3:w423:path)  [unwired: 3 in, 2 out]
                n207 = Unbundle(w417) -> ()  [unwired: 3 out]
                n208 = Path To String(path=w423) -> (string=w422:string)
                n209 = Bundle By Name(cluster=T8 {"Command"="", "Parameter"=""} ("element"), "Command"="OPEN_FITS_FILE", "Parameter"=w422) -> (w419:T8)
                n210 = Enqueue Element(queue=w420, element=w419, error in (no error)=w421) -> ()  [unwired: 1 in, 3 out]
              }
              frame False {
              }
            }
          }
          event "Image Open 2": Mouse Down {
            n211 = event-data() -> ()  [unwired: 1 in, 8 out]
            n212 = case shown="True" "Image Open 2" {
              tunnel: w430 -> [w436 _]
              tunnel: w431 -> [w435 _]
              frame True {
                (unwired) T9."existing file" ("select mode (2)")
                n213 = File Dialog(5:"Open Image" ("button label"), 6:"*.fits" ("default name"), 7:"Open Image" ("prompt"), 11:path "C:/DATA" ("start path")) -> (0:w432:errorcluster, 3:w438:path)  [unwired: 3 in, 2 out]
                n214 = Unbundle(w432) -> ()  [unwired: 3 out]
                n215 = Path To String(path=w438) -> (string=w437:string)
                n216 = Bundle By Name(cluster=T8 {"Command"="", "Parameter"=""} ("element"), "Command"="OPEN_FITS_FILE", "Parameter"=w437) -> (w434:T8)
                n217 = Enqueue Element(queue=w435, element=w434, error in (no error)=w436) -> ()  [unwired: 1 in, 3 out]
              }
              frame False {
              }
            }
          }
          event "Redraw 2": Mouse Down {
            n218 = event-data() -> ()  [unwired: 1 in, 8 out]
            n219 = Enqueue Element(queue=w445, element=T8 {"Command"="DISPLAY_IMAGE", "Parameter"=""}, error in (no error)=w444) -> ()  [unwired: 1 in, 3 out]
          }
          event Key Down {
            n220 = event-data() -> ("Char"=w449:i16)  [unwired: 1 in]
            n221 = case shown="\"Slits\"" w453 {
              tunnel: w452 -> [w459 w618]
              tunnel: w451 -> [w458 w619]
              tunnel: w450 -> [w457 w614]
              tunnel: w449 -> [w456 w615]
              tunnel: w448 -> [w455 w617]
              tunnel: w447 -> [w454 w616]
              frame "Stars", Default {
                n222 = case shown="114" w456 {
                  selector: w456 -> [_ _ _ _ w528 _ _ _ _]
                  tunnel: w459 -> [_ w460 _ _ w524 w547 _ _ _]
                  tunnel: w458 -> [_ w461 _ _ w523 w548 _ _ _]
                  tunnel: w457 -> [_ _ _ _ _ _ _ _ _]
                  tunnel: w455 -> [_ _ _ _ _ _ _ _ _]
                  tunnel: w454 -> [_ _ _ _ _ _ _ _ _]
                  frame 0 {
                  }
                  frame 97 {
                    n223 = local read "Zoom Window"() -> (w462:i16[][])
                    n224 = Array Size(array=w462) -> (size(s)=w466:i32[])
                    n225 = Index Array(array=w466, index=1) -> (element=w467:i32)
                    n226 = Index Array(array=w466, index=0) -> (element=w464:i32)
                    n227 = stacked-sequence {
                      seq-local: [w470 _ _] -> [_ w482 _]
                      seq-local: [_ w487 _] -> [_ _ w500]
                      tunnel: w462 -> [w474 _ _]
                      tunnel: w464 -> [w468 _ _]
                      tunnel: w467 -> [w469 _ _]
                      tunnel: w461 -> [_ _ w497]
                      tunnel: w460 -> [_ _ w498]
                      frame #0 {
                        n228 = Initialize Array(0 ("element"), w468) -> (w473:i32[])
                        n229 = for {
                          N: w469 -> [_]
                          tunnel: w474 -> [w480]
                          shift-right: [w479] -> w471
                          shift-left: w473 -> [w477]
                          i -> [w475]
                          n230 = Index Array(array=w480, index (col)=w475) -> (element=w478:i16[])  [unwired: 1 in]
                          n231 = Add(x=w478, y=w477) -> (x+y=w476:i32[])
                          n232 = Replace Array Subset(array=w477, new element=w476) -> (w479:i32[])  [unwired: 1 in]
                        }
                        n233 = Array Max & Min(array=w471) -> (max index (indices)=w470:i32)  [unwired: 3 out]
                      }
                      frame #1 {
                        n234 = property on="Zoom Window" class="IntGraph (strict)"() -> ("X Scale.Range:Minimum"=w485:dbl)  [unwired: 2 in, 2 out]
                        n235 = property on="Zoom Window" class="IntGraph (strict)"() -> ("X Scale.Range:Maximum"=w486:dbl)  [unwired: 2 in, 2 out]
                        n236 = Subtract(x=w486, y=w485) -> (x-y=w484:dbl)
                        n237 = Divide(x=w484, y=2) -> (x/y=w489:dbl)
                        n238 = Decrement(x=w482) -> (x-1=w481:i32)
                        n239 = local read "X"() -> (w483:dbl)
                        n240 = Subtract(x=w481, y=w489) -> (x-y=w488:dbl)
                        n241 = Add(x=w488, y=w483) -> (x+y=w487:dbl)
                      }
                      frame #2 {
                        n242 = local read "Display Binning"() -> (w494:i16)
                        n243 = Enqueue Element(queue=w497, element=T8 {"Command"="UPDATE_ZOOM", "Parameter"=""}, error in (no error)=w498) -> ()  [unwired: 1 in, 3 out]
                        n244 = Equal To 0?(x=w494) -> (x = 0?=w495:bool)
                        n245 = Select(t=u16 1, s=w495, f=w494) -> (s? t:f=w492:u16)
                        n246 = To Double Precision Float(number=w492) -> (double precision float=w493:dbl)
                        n247 = Divide(x=w500, y=w493) -> (x/y=w491:dbl)
                        n248 = property on="Image1" class="IntGraph (strict)"("Cursor.Cursor Position:Cursor X"=w491) -> ()  [unwired: 2 in, 2 out]
                      }
                    }
                  }
                  frame 99 {
                    n249 = property on="Image1" class="IntGraph (strict)"() -> ("X Scale.Range:Maximum"=w512:dbl)  [unwired: 2 in, 2 out]
                    n250 = property on="Image1" class="IntGraph (strict)"() -> ("X Scale.Range:Minimum"=w503:dbl)  [unwired: 2 in, 2 out]
                    n251 = property on="Image1" class="IntGraph (strict)"() -> ("Y Scale.Range:Maximum"=w513:dbl)  [unwired: 2 in, 2 out]
                    n252 = property on="Image1" class="IntGraph (strict)"() -> ("Y Scale.Range:Minimum"=w507:dbl)  [unwired: 2 in, 2 out]
                    n253 = Subtract(x=w513, y=w507) -> (x-y=w509:dbl)
                    n254 = Subtract(x=w512, y=w503) -> (x-y=w504:dbl)
                    n255 = Divide(x=w509, y=2) -> (x/y=w508:dbl)
                    n256 = Divide(x=w504, y=2) -> (x/y=w505:dbl)
                    n257 = Add(x=w508, y=w507) -> (x+y=w501:dbl)
                    n258 = Add(x=w505, y=w503) -> (x+y=w502:dbl)
                    n259 = Bundle(w502, w501) -> (w511:cluster{dbl, dbl})  [unwired: 1 in]
                    n260 = property on="Image1" class="IntGraph (strict)"("Cursor.Cursor Position"=w511) -> ()  [unwired: 2 in, 2 out]
                  }
                  frame 104 {
                    n261 = local write "Tab Control"(T4."FITS Headers" ("Tab Control")) -> ()
                  }
                  frame 105..108 {
                    n262 = property on="Image1" class="IntGraph (strict)"() -> ("Cursor.Cursor Position:Cursor X"=w520:dbl)  [unwired: 2 in, 2 out]
                    n263 = property on="Image1" class="IntGraph (strict)"() -> ("Cursor.Cursor Position:Cursor Y"=w519:dbl)  [unwired: 2 in, 2 out]
                    n264 = Enqueue Element(queue=w523, element=T8 {"Command"="UPDATE_ZOOM", "Parameter"=""}, error in (no error)=w524) -> ()  [unwired: 1 in, 3 out]
                    n265 = local read "Display Binning"() -> (w516:i16)
                    n266 = Equal To 0?(x=w516) -> (x = 0?=w518:bool)
                    n267 = Select(t=i8 1, s=w518, f=w516) -> (s? t:f=w515:i16)
                    n268 = Divide(x=u16 1 ("t"), y=w515) -> (x/y=w521:dbl)
                    n269 = case shown="107" w528 {
                      tunnel: w520 -> [w530 w533 w538 w541 w546]
                      tunnel: [w530 w532 w538 w540 w546] -> w527
                      tunnel: w519 -> [w529 w534 w536 w542 w544]
                      tunnel: [w529 w534 w535 w542 w543] -> w526
                      tunnel: w521 -> [_ w531 w537 w539 w545]
                      frame 0, Default {
                      }
                      frame 108 {
                        n270 = Add(x=w533, y=w531) -> (x+y=w532:dbl)
                      }
                      frame 105 {
                        n271 = Add(x=w536, y=w537) -> (x+y=w535:dbl)
                      }
                      frame 106 {
                        n272 = Subtract(x=w541, y=w539) -> (x-y=w540:dbl)
                      }
                      frame 107 {
                        n273 = Subtract(x=w544, y=w545) -> (x-y=w543:dbl)
                      }
                    }
                    n274 = property on="Image1" class="IntGraph (strict)"("Cursor.Cursor Position:Cursor X"=w527) -> ()  [unwired: 2 in, 2 out]
                    n275 = property on="Image1" class="IntGraph (strict)"("Cursor.Cursor Position:Cursor Y"=w526) -> ()  [unwired: 2 in, 2 out]
                  }
                  frame 114 {
                    n276 = local read "Zoom Window"() -> (w554:i16[][])
                    n277 = Array Size(array=w554) -> (size(s)=w550:i32[])
                    n278 = Index Array(array=w550, index=1) -> (element=w549:i32)
                    n279 = Index Array(array=w550, index=0) -> (element=w552:i32)
                    n280 = stacked-sequence {
                      seq-local: [w555 _ _ _] -> [_ _ w593 _]
                      seq-local: [_ w568 _ _] -> [_ _ w594 _]
                      seq-local: [_ _ w581 _] -> [_ _ _ w612]
                      tunnel: w554 -> [w561 w572 _ _]
                      tunnel: w552 -> [w558 w571 _ _]
                      tunnel: w549 -> [w557 w570 _ _]
                      tunnel: w548 -> [_ _ _ w608]
                      tunnel: w547 -> [_ _ _ w607]
                      frame #0 {
                        n281 = Initialize Array(0 ("element"), w557) -> (w560:i32[])
                        n282 = for {
                          N: w558 -> [_]
                          tunnel: w561 -> [w567]
                          shift-right: [w566] -> w556
                          shift-left: w560 -> [w564]
                          i -> [w562]
                          n283 = Index Array(array=w567, index (row)=w562) -> (element=w565:i16[])  [unwired: 1 in]
                          n284 = Add(x=w565, y=w564) -> (x+y=w563:i32[])
                          n285 = Replace Array Subset(array=w564, new element=w563) -> (w566:i32[])  [unwired: 1 in]
                        }
                        n286 = Array Max & Min(array=w556) -> (max index (indices)=w555:i32)  [unwired: 3 out]
                      }
                      frame #1 {
                        n287 = Initialize Array(0 ("element"), w571) -> (w574:i32[])
                        n288 = for {
                          N: w570 -> [_]
                          tunnel: w572 -> [w580]
                          shift-right: [w579] -> w569
                          shift-left: w574 -> [w576]
                          i -> [w575]
                          n289 = Index Array(array=w580, index (col)=w575) -> (element=w577:i16[])  [unwired: 1 in]
                          n290 = Add(x=w577, y=w576) -> (x+y=w578:i32[])
                          n291 = Replace Array Subset(array=w576, new element=w578) -> (w579:i32[])  [unwired: 1 in]
                        }
                        n292 = Array Max & Min(array=w569) -> (max index (indices)=w568:i32)  [unwired: 3 out]
                      }
                      frame #2 {
                        n293 = property on="Zoom Window" class="IntGraph (strict)"() -> ("Y Scale.Range:Minimum"=w586:dbl)  [unwired: 2 in, 2 out]
                        n294 = property on="Zoom Window" class="IntGraph (strict)"() -> ("X Scale.Range:Maximum"=w588:dbl)  [unwired: 2 in, 2 out]
                        n295 = property on="Zoom Window" class="IntGraph (strict)"() -> ("X Scale.Range:Minimum"=w589:dbl)  [unwired: 2 in, 2 out]
                        n296 = property on="Zoom Window" class="IntGraph (strict)"() -> ("Y Scale.Range:Maximum"=w587:dbl)  [unwired: 2 in, 2 out]
                        n297 = Subtract(x=w588, y=w589) -> (x-y=w591:dbl)
                        n298 = Subtract(x=w587, y=w586) -> (x-y=w592:dbl)
                        n299 = Bundle(w591, w592) -> (w595:cluster{dbl, dbl})  [unwired: 1 in]
                        n300 = local read "X"() -> (w599:dbl)
                        n301 = local read "Y"() -> (w598:dbl)
                        n302 = Divide(x=w595, y=2) -> (x/y=w590:cluster{dbl, dbl})
                        n303 = Bundle(w594, w593) -> (w597:cluster{i32, i32})  [unwired: 1 in]
                        n304 = Bundle("X"=w599, "Y"=w598) -> (w596:cluster{"X":dbl, "Y":dbl})  [unwired: 1 in]
                        n305 = Subtract(x=w597, y=w590) -> (x-y=w584:cluster{dbl, dbl})
                        n306 = To Word Integer(number=w584) -> (16bit integer=w585:cluster{i16, i16})
                        n307 = To Double Precision Float(number=w585) -> (double precision float=w583:cluster{dbl, dbl})
                        n308 = Add(x=w583, y=w596) -> (x+y=w582:cluster{dbl, dbl})
                        n309 = To Word Integer(number=w582) -> (16bit integer=w581:cluster{i16, i16})
                      }
                      frame #3 {
                        n310 = Enqueue Element(queue=w608, element=T8 {"Command"="ZOOM_FOR_GAUSS_FIT", "Parameter"=""}, error in (no error)=w607) -> (queue out=w605:refnum<queue>, error out=w606:errorcluster)  [unwired: 1 in, 1 out]
                        n311 = local read "Display Binning"() -> (w601:i16)
                        n312 = Enqueue Element(queue=w605, element=T8 {"Command"="FIT_GAUSSIAN", "Parameter"=""}, error in (no error)=w606) -> ()  [unwired: 1 in, 3 out]
                        n313 = Equal To 0?(x=w601) -> (x = 0?=w603:bool)
                        n314 = Select(t=u16 1, s=w603, f=w601) -> (s? t:f=w602:u16)
                        n315 = Divide(x=w612, y=w602) -> (x/y=w611:cluster{dbl, dbl})
                        n316 = property on="Image1" class="IntGraph (strict)"("Cursor.Cursor Position"=w611) -> ()  [unwired: 2 in, 2 out]
                      }
                    }
                  }
                  frame 115 {
                  }
                  frame 116 {
                    n317 = local write "Tab Control"(T4."Stars" ("Tab Control")) -> ()
                  }
                  frame Default {
                  }
                }
              }
              frame "Slits" {
                n318 = case shown="99" w615 {
                  selector: w615 -> [_ _ _ _ w688 _ _ _ _]
                  tunnel: w618 -> [_ w621 _ _ w686 w708 _ _ _]
                  tunnel: w619 -> [_ w622 _ _ w685 w709 _ _ _]
                  tunnel: w617 -> [_ _ _ _ _ _ _ _ _]
                  tunnel: w616 -> [_ _ _ _ _ _ _ _ _]
                  tunnel: w614 -> [_ _ _ _ _ _ _ _ _]
                  frame 0 {
                  }
                  frame 97 {
                    n319 = local read "Zoom Window 2"() -> (w620:i16[][])
                    n320 = Array Size(array=w620) -> (size(s)=w626:i32[])
                    n321 = Index Array(array=w626, index=1) -> (element=w627:i32)
                    n322 = Index Array(array=w626, index=0) -> (element=w624:i32)
                    n323 = stacked-sequence {
                      seq-local: [w630 _ _] -> [_ w645 _]
                      seq-local: [_ w647 _] -> [_ _ w660]
                      tunnel: w620 -> [w634 _ _]
                      tunnel: w624 -> [w628 _ _]
                      tunnel: w627 -> [w629 _ _]
                      tunnel: w622 -> [_ _ w657]
                      tunnel: w621 -> [_ _ w658]
                      frame #0 {
                        n324 = Initialize Array(0 ("element"), w628) -> (w633:i32[])
                        n325 = for {
                          N: w629 -> [_]
                          tunnel: w634 -> [w640]
                          shift-right: [w639] -> w631
                          shift-left: w633 -> [w637]
                          i -> [w635]
                          n326 = Index Array(array=w640, index (col)=w635) -> (element=w638:i16[])  [unwired: 1 in]
                          n327 = Add(x=w638, y=w637) -> (x+y=w636:i32[])
                          n328 = Replace Array Subset(array=w637, new element=w636) -> (w639:i32[])  [unwired: 1 in]
                        }
                        n329 = Array Max & Min(array=w631) -> (max index (indices)=w630:i32)  [unwired: 3 out]
                      }
                      frame #1 {
                        n330 = property on="Zoom Window 2" class="IntGraph (strict)"() -> ("X Scale.Range:Maximum"=w643:dbl)  [unwired: 2 in, 2 out]
                        n331 = property on="Zoom Window 2" class="IntGraph (strict)"() -> ("X Scale.Range:Minimum"=w642:dbl)  [unwired: 2 in, 2 out]
                        n332 = Subtract(x=w643, y=w642) -> (x-y=w646:dbl)
                        n333 = Divide(x=w646, y=2) -> (x/y=w649:dbl)
                        n334 = local read "X 2"() -> (w641:dbl)
                        n335 = Decrement(x=w645) -> (x-1=w644:i32)
                        n336 = Subtract(x=w644, y=w649) -> (x-y=w648:dbl)
                        n337 = Add(x=w648, y=w641) -> (x+y=w647:dbl)
                      }
                      frame #2 {
                        n338 = local read "Display Binning 2"() -> (w651:i16)
                        n339 = Enqueue Element(queue=w657, element=T8 {"Command"="UPDATE_ZOOM", "Parameter"=""}, error in (no error)=w658) -> ()  [unwired: 1 in, 3 out]
                        n340 = Equal To 0?(x=w651) -> (x = 0?=w655:bool)
                        n341 = Select(t=u16 1, s=w655, f=w651) -> (s? t:f=w653:u16)
                        n342 = To Double Precision Float(number=w653) -> (double precision float=w654:dbl)
                        n343 = Divide(x=w660, y=w654) -> (x/y=w652:dbl)
                        n344 = property on="Image2" class="IntGraph (strict)"("Cursor.Cursor Position:Cursor X"=w652) -> ()  [unwired: 2 in, 2 out]
                      }
                    }
                  }
                  frame 99 {
                    n345 = property on="Image2" class="IntGraph (strict)"() -> ("Y Scale.Range:Maximum"=w663:dbl)  [unwired: 2 in, 2 out]
                    n346 = property on="Image2" class="IntGraph (strict)"() -> ("X Scale.Range:Maximum"=w665:dbl)  [unwired: 2 in, 2 out]
                    n347 = property on="Image2" class="IntGraph (strict)"() -> ("Y Scale.Range:Minimum"=w662:dbl)  [unwired: 2 in, 2 out]
                    n348 = property on="Image2" class="IntGraph (strict)"() -> ("X Scale.Range:Minimum"=w664:dbl)  [unwired: 2 in, 2 out]
                    n349 = Subtract(x=w663, y=w662) -> (x-y=w672:dbl)
                    n350 = Subtract(x=w665, y=w664) -> (x-y=w668:dbl)
                    n351 = Divide(x=w672, y=2) -> (x/y=w671:dbl)
                    n352 = Divide(x=w668, y=2) -> (x/y=w669:dbl)
                    n353 = Add(x=w671, y=w662) -> (x+y=w666:dbl)
                    n354 = Add(x=w669, y=w664) -> (x+y=w667:dbl)
                    n355 = Bundle(w667, w666) -> (w661:cluster{dbl, dbl})  [unwired: 1 in]
                    n356 = property on="Image2" class="IntGraph (strict)"("Cursor.Cursor Position"=w661) -> ()  [unwired: 2 in, 2 out]
                  }
                  frame 104 {
                    n357 = local write "Tab Control"(T4."FITS Headers" ("Tab Control")) -> ()
                  }
                  frame 105..108 {
                    n358 = property on="Image2" class="IntGraph (strict)"() -> ("Cursor.Cursor Position:Cursor X"=w678:dbl)  [unwired: 2 in, 2 out]
                    n359 = property on="Image2" class="IntGraph (strict)"() -> ("Cursor.Cursor Position:Cursor Y"=w677:dbl)  [unwired: 2 in, 2 out]
                    n360 = Enqueue Element(queue=w685, element=T8 {"Command"="UPDATE_ZOOM", "Parameter"=""}, error in (no error)=w686) -> ()  [unwired: 1 in, 3 out]
                    n361 = local read "Display Binning 2"() -> (w679:i16)
                    n362 = Equal To 0?(x=w679) -> (x = 0?=w682:bool)
                    n363 = Select(t=i8 1, s=w682, f=w679) -> (s? t:f=w680:i16)
                    n364 = Divide(x=u16 1 ("t"), y=w680) -> (x/y=w683:dbl)
                    n365 = case shown="106" w688 {
                      tunnel: w678 -> [w690 w693 w698 w701 w706]
                      tunnel: [w690 w692 w698 w700 w706] -> w676
                      tunnel: w677 -> [w689 w694 w696 w702 w704]
                      tunnel: [w689 w694 w695 w702 w703] -> w675
                      tunnel: w683 -> [_ w691 w697 w699 w705]
                      frame 0, Default {
                      }
                      frame 108 {
                        n366 = Add(x=w693, y=w691) -> (x+y=w692:dbl)
                      }
                      frame 105 {
                        n367 = Add(x=w696, y=w697) -> (x+y=w695:dbl)
                      }
                      frame 106 {
                        n368 = Subtract(x=w701, y=w699) -> (x-y=w700:dbl)
                      }
                      frame 107 {
                        n369 = Subtract(x=w704, y=w705) -> (x-y=w703:dbl)
                      }
                    }
                    n370 = property on="Image2" class="IntGraph (strict)"("Cursor.Cursor Position:Cursor X"=w676) -> ()  [unwired: 2 in, 2 out]
                    n371 = property on="Image2" class="IntGraph (strict)"("Cursor.Cursor Position:Cursor Y"=w675) -> ()  [unwired: 2 in, 2 out]
                  }
                  frame 114 {
                    n372 = local read "Zoom Window 2"() -> (w707:i16[][])
                    n373 = Array Size(array=w707) -> (size(s)=w711:i32[])
                    n374 = Index Array(array=w711, index=1) -> (element=w710:i32)
                    n375 = Index Array(array=w711, index=0) -> (element=w713:i32)
                    n376 = stacked-sequence {
                      seq-local: [w715 _ _ _] -> [_ _ w755 _]
                      seq-local: [_ w728 _ _] -> [_ _ w756 _]
                      seq-local: [_ _ w747 _] -> [_ _ _ w772]
                      tunnel: w707 -> [w721 w732 _ _]
                      tunnel: w713 -> [w718 w731 _ _]
                      tunnel: w710 -> [w717 w730 _ _]
                      tunnel: w709 -> [_ _ _ w769]
                      tunnel: w708 -> [_ _ _ w768]
                      frame #0 {
                        n377 = Initialize Array(0 ("element"), w717) -> (w720:i32[])
                        n378 = for {
                          N: w718 -> [_]
                          tunnel: w721 -> [w727]
                          shift-right: [w726] -> w716
                          shift-left: w720 -> [w724]
                          i -> [w722]
                          n379 = Index Array(array=w727, index (row)=w722) -> (element=w725:i16[])  [unwired: 1 in]
                          n380 = Add(x=w725, y=w724) -> (x+y=w723:i32[])
                          n381 = Replace Array Subset(array=w724, new element=w723) -> (w726:i32[])  [unwired: 1 in]
                        }
                        n382 = Array Max & Min(array=w716) -> (max index (indices)=w715:i32)  [unwired: 3 out]
                      }
                      frame #1 {
                        n383 = Initialize Array(0 ("element"), w731) -> (w734:i32[])
                        n384 = for {
                          N: w730 -> [_]
                          tunnel: w732 -> [w740]
                          shift-right: [w739] -> w729
                          shift-left: w734 -> [w736]
                          i -> [w735]
                          n385 = Index Array(array=w740, index (col)=w735) -> (element=w737:i16[])  [unwired: 1 in]
                          n386 = Add(x=w737, y=w736) -> (x+y=w738:i32[])
                          n387 = Replace Array Subset(array=w736, new element=w738) -> (w739:i32[])  [unwired: 1 in]
                        }
                        n388 = Array Max & Min(array=w729) -> (max index (indices)=w728:i32)  [unwired: 3 out]
                      }
                      frame #2 {
                        n389 = property on="Zoom Window 2" class="IntGraph (strict)"() -> ("X Scale.Range:Maximum"=w744:dbl)  [unwired: 2 in, 2 out]
                        n390 = property on="Zoom Window 2" class="IntGraph (strict)"() -> ("Y Scale.Range:Maximum"=w742:dbl)  [unwired: 2 in, 2 out]
                        n391 = property on="Zoom Window 2" class="IntGraph (strict)"() -> ("X Scale.Range:Minimum"=w743:dbl)  [unwired: 2 in, 2 out]
                        n392 = property on="Zoom Window 2" class="IntGraph (strict)"() -> ("Y Scale.Range:Minimum"=w741:dbl)  [unwired: 2 in, 2 out]
                        n393 = Subtract(x=w744, y=w743) -> (x-y=w753:dbl)
                        n394 = Subtract(x=w742, y=w741) -> (x-y=w754:dbl)
                        n395 = Bundle(w753, w754) -> (w757:cluster{dbl, dbl})  [unwired: 1 in]
                        n396 = local read "Y 2"() -> (w745:dbl)
                        n397 = local read "X 2"() -> (w746:dbl)
                        n398 = Divide(x=w757, y=2) -> (x/y=w752:cluster{dbl, dbl})
                        n399 = Bundle(w756, w755) -> (w759:cluster{i32, i32})  [unwired: 1 in]
                        n400 = Bundle("X 2"=w746, "Y 2"=w745) -> (w758:cluster{"X 2":dbl, "Y 2":dbl})  [unwired: 1 in]
                        n401 = Subtract(x=w759, y=w752) -> (x-y=w750:cluster{dbl, dbl})
                        n402 = To Word Integer(number=w750) -> (16bit integer=w751:cluster{i16, i16})
                        n403 = To Double Precision Float(number=w751) -> (double precision float=w749:cluster{dbl, dbl})
                        n404 = Add(x=w749, y=w758) -> (x+y=w748:cluster{dbl, dbl})
                        n405 = To Word Integer(number=w748) -> (16bit integer=w747:cluster{i16, i16})
                      }
                      frame #3 {
                        n406 = Enqueue Element(queue=w769, element=T8 {"Command"="ZOOM_FOR_GAUSS_FIT", "Parameter"=""}, error in (no error)=w768) -> (queue out=w766:refnum<queue>, error out=w767:errorcluster)  [unwired: 1 in, 1 out]
                        n407 = local read "Display Binning 2"() -> (w762:i16)
                        n408 = Enqueue Element(queue=w766, element=T8 {"Command"="FIT_GAUSSIAN", "Parameter"=""}, error in (no error)=w767) -> ()  [unwired: 1 in, 3 out]
                        n409 = Equal To 0?(x=w762) -> (x = 0?=w764:bool)
                        n410 = Select(t=u16 1, s=w764, f=w762) -> (s? t:f=w763:u16)
                        n411 = Divide(x=w772, y=w763) -> (x/y=w761:cluster{dbl, dbl})
                        n412 = property on="Image2" class="IntGraph (strict)"("Cursor.Cursor Position"=w761) -> ()  [unwired: 2 in, 2 out]
                      }
                    }
                  }
                  frame 115 {
                  }
                  frame 116 {
                    n413 = local write "Tab Control"(T4."Stars" ("Tab Control")) -> ()
                  }
                  frame Default {
                  }
                }
              }
            }
          }
          event "Send Target Offset Position": Value Change {
            w783 = " " ("string")
            n414 = event-data() -> ()  [unwired: 1 in, 1 out]
            n415 = local read "Offsets and Rotation"() -> (w777:T7)
            n416 = Unbundle By Name(w777) -> ("Delta X"=w776:dbl, "Delta Y"=w775:dbl)
            n417 = Format Into String(w776) -> (resulting string=w789:string)  [unwired: 3 in, 1 out]
            n418 = Format Into String(w775) -> (resulting string=w788:string)  [unwired: 3 in, 1 out]
            n419 = Obtain Queue(name (unnamed)="SICAMERA_Command_Q", element data type=T8 {"Command"="", "Parameter"=""} ("element")) -> (queue out=w781:refnum<queue>, created new?=w780:bool, error out=w779:errorcluster)  [unwired: 3 in]
            n420 = Concatenate Strings("T" ("string"), w783, w789, w783, w788) -> (w786:string)
            n421 = Bundle("Command"="ACCEPT_OFFSET_COORD", w786) -> (w778:cluster{"Command":string, string})  [unwired: 1 in]
            n422 = case shown="False" w780 {
              tunnel: w778 -> [_ w799]
              tunnel: w781 -> [w791 w798]
              tunnel: w779 -> [w792 w797]
              tunnel: ["Error upon sending the offset coord." ("Image Status") "Coordinates successfully uploaded to GSCS!" ("Image Status")] -> w774
              frame True {
                n423 = Release Queue(queue=w791, error in (no error)=w792) -> ()  [unwired: 1 in, 3 out]
              }
              frame False {
                n424 = Enqueue Element(queue=w798, element=w799, error in (no error)=w797) -> (queue out=w796:refnum<queue>, error out=w795:errorcluster)  [unwired: 1 in, 1 out]
                n425 = Release Queue(queue=w796, error in (no error)=w795) -> ()  [unwired: 1 in, 3 out]
              }
            }
            "String 3" <- w774
            n426 = local write "Send Target Offset Position"(FALSE ("Send Target Offset Position")) -> ()
          }
          event "Zoom In": Mouse Down {
            n427 = event-data() -> ()  [unwired: 1 in, 8 out]
            n428 = property on="Image1" class="IntGraph (strict)"() -> ("X Scale.Range"=w807:T10)  [unwired: 2 in, 2 out]
            n429 = property on="Image1" class="IntGraph (strict)"() -> ("Y Scale.Range"=w802:T10)  [unwired: 2 in, 2 out]
            n430 = Unbundle By Name(w807) -> ("Maximum"=w821:dbl, "Minimum"=w815:dbl)
            n431 = Unbundle By Name(w802) -> ("Maximum"=w814:dbl, "Minimum"=w809:dbl)
            n432 = Subtract(x=w821, y=w815) -> (x-y=w820:dbl)
            n433 = Subtract(x=w814, y=w809) -> (x-y=w819:dbl)
            n434 = Bundle(w820, w819) -> (w816:cluster{dbl, dbl})  [unwired: 1 in]
            n435 = Bundle("Minimum"=w815, "Minimum"=w809) -> (w812:cluster{"Minimum":dbl, "Minimum":dbl})  [unwired: 1 in]
            n436 = Multiply(x=w816, y=0.5) -> (x*y=w810:cluster{dbl, dbl})
            n437 = Multiply(x=w816, y=0.25) -> (x*y=w813:cluster{dbl, dbl})
            n438 = Add(x=w813, y=w812) -> (x+y=w811:cluster{dbl, dbl})
            n439 = Add(x=w810, y=w811) -> (x+y=w806:cluster{dbl, dbl})
            n440 = Unbundle(w811) -> (w804:dbl, w801:dbl)
            n441 = Unbundle(w806) -> (w805:dbl, w800:dbl)
            n442 = Bundle By Name(cluster=w802, "Maximum"=w800, "Minimum"=w801) -> (w803:T10)
            n443 = Bundle By Name(cluster=w807, "Maximum"=w805, "Minimum"=w804) -> (w808:T10)
            n444 = property on="Image1" class="IntGraph (strict)"("Y Scale.Range"=w803) -> ()  [unwired: 2 in, 2 out]
            n445 = property on="Image1" class="IntGraph (strict)"("X Scale.Range"=w808) -> ()  [unwired: 2 in, 2 out]
          }
          event "Zoom In 2": Mouse Down {
            n446 = event-data() -> ()  [unwired: 1 in, 8 out]
            n447 = property on="Image2" class="IntGraph (strict)"() -> ("Y Scale.Range"=w824:T10)  [unwired: 2 in, 2 out]
            n448 = property on="Image2" class="IntGraph (strict)"() -> ("X Scale.Range"=w825:T10)  [unwired: 2 in, 2 out]
            n449 = Unbundle By Name(w825) -> ("Maximum"=w843:dbl, "Minimum"=w837:dbl)
            n450 = Unbundle By Name(w824) -> ("Maximum"=w836:dbl, "Minimum"=w831:dbl)
            n451 = Subtract(x=w843, y=w837) -> (x-y=w842:dbl)
            n452 = Subtract(x=w836, y=w831) -> (x-y=w841:dbl)
            n453 = Bundle(w842, w841) -> (w838:cluster{dbl, dbl})  [unwired: 1 in]
            n454 = Bundle("Minimum"=w837, "Minimum"=w831) -> (w834:cluster{"Minimum":dbl, "Minimum":dbl})  [unwired: 1 in]
            n455 = Multiply(x=w838, y=0.5) -> (x*y=w832:cluster{dbl, dbl})
            n456 = Multiply(x=w838, y=0.25) -> (x*y=w835:cluster{dbl, dbl})
            n457 = Add(x=w835, y=w834) -> (x+y=w833:cluster{dbl, dbl})
            n458 = Add(x=w832, y=w833) -> (x+y=w830:cluster{dbl, dbl})
            n459 = Unbundle(w833) -> (w828:dbl, w827:dbl)
            n460 = Unbundle(w830) -> (w829:dbl, w826:dbl)
            n461 = Bundle By Name(cluster=w824, "Maximum"=w826, "Minimum"=w827) -> (w822:T10)
            n462 = Bundle By Name(cluster=w825, "Maximum"=w829, "Minimum"=w828) -> (w823:T10)
            n463 = property on="Image2" class="IntGraph (strict)"("Y Scale.Range"=w822) -> ()  [unwired: 2 in, 2 out]
            n464 = property on="Image2" class="IntGraph (strict)"("X Scale.Range"=w823) -> ()  [unwired: 2 in, 2 out]
          }
          event "Zoom Out": Mouse Down {
            n465 = event-data() -> ()  [unwired: 1 in, 8 out]
            n466 = property on="Image1" class="IntGraph (strict)"() -> ("X Scale.Range"=w863:T10)  [unwired: 2 in, 2 out]
            n467 = property on="Image1" class="IntGraph (strict)"() -> ("Y Scale.Range"=w862:T10)  [unwired: 2 in, 2 out]
            n468 = Unbundle By Name(w863) -> ("Maximum"=w861:dbl, "Minimum"=w855:dbl)
            n469 = Unbundle By Name(w862) -> ("Maximum"=w854:dbl, "Minimum"=w847:dbl)
            n470 = Subtract(x=w861, y=w855) -> (x-y=w860:dbl)
            n471 = Subtract(x=w854, y=w847) -> (x-y=w859:dbl)
            n472 = Bundle(w860, w859) -> (w856:cluster{dbl, dbl})  [unwired: 1 in]
            n473 = Bundle("Minimum"=w855, "Minimum"=w847) -> (w845:cluster{"Minimum":dbl, "Minimum":dbl})  [unwired: 1 in]
            n474 = Multiply(x=w856, y=2) -> (x*y=w846:cluster{dbl, dbl})
            n475 = Multiply(x=w846, y=0.25) -> (x*y=w844:cluster{dbl, dbl})
            n476 = Subtract(x=w845, y=w844) -> (x-y=w853:cluster{dbl, dbl})
            n477 = Add(x=w846, y=w853) -> (x+y=w850:cluster{dbl, dbl})
            n478 = Unbundle(w853) -> (w852:dbl, w851:dbl)
            n479 = Unbundle(w850) -> (w849:dbl, w848:dbl)
            n480 = property on="Image1" class="IntGraph (strict)"("Y Scale.Range:Minimum"=w851) -> ()  [unwired: 2 in, 2 out]
            n481 = property on="Image1" class="IntGraph (strict)"("X Scale.Range:Minimum"=w852) -> ()  [unwired: 2 in, 2 out]
            n482 = property on="Image1" class="IntGraph (strict)"("X Scale.Range:Maximum"=w849) -> ()  [unwired: 2 in, 2 out]
            n483 = property on="Image1" class="IntGraph (strict)"("Y Scale.Range:Maximum"=w848) -> ()  [unwired: 2 in, 2 out]
          }
          event "Zoom Out 2": Mouse Down {
            n484 = event-data() -> ()  [unwired: 1 in, 8 out]
            n485 = property on="Image2" class="IntGraph (strict)"() -> ("X Scale.Range"=w869:T10)  [unwired: 2 in, 2 out]
            n486 = property on="Image2" class="IntGraph (strict)"() -> ("Y Scale.Range"=w868:T10)  [unwired: 2 in, 2 out]
            n487 = Unbundle By Name(w869) -> ("Maximum"=w883:dbl, "Minimum"=w877:dbl)
            n488 = Unbundle By Name(w868) -> ("Maximum"=w876:dbl, "Minimum"=w873:dbl)
            n489 = Subtract(x=w883, y=w877) -> (x-y=w882:dbl)
            n490 = Subtract(x=w876, y=w873) -> (x-y=w881:dbl)
            n491 = Bundle(w882, w881) -> (w878:cluster{dbl, dbl})  [unwired: 1 in]
            n492 = Bundle("Minimum"=w877, "Minimum"=w873) -> (w871:cluster{"Minimum":dbl, "Minimum":dbl})  [unwired: 1 in]
            n493 = Multiply(x=w878, y=2) -> (x*y=w872:cluster{dbl, dbl})
            n494 = Multiply(x=w872, y=0.25) -> (x*y=w870:cluster{dbl, dbl})
            n495 = Subtract(x=w871, y=w870) -> (x-y=w875:cluster{dbl, dbl})
            n496 = Add(x=w872, y=w875) -> (x+y=w874:cluster{dbl, dbl})
            n497 = Unbundle(w875) -> (w865:dbl, w864:dbl)
            n498 = Unbundle(w874) -> (w867:dbl, w866:dbl)
            n499 = property on="Image2" class="IntGraph (strict)"("X Scale.Range:Minimum"=w865) -> ()  [unwired: 2 in, 2 out]
            n500 = property on="Image2" class="IntGraph (strict)"("Y Scale.Range:Minimum"=w864) -> ()  [unwired: 2 in, 2 out]
            n501 = property on="Image2" class="IntGraph (strict)"("X Scale.Range:Maximum"=w867) -> ()  [unwired: 2 in, 2 out]
            n502 = property on="Image2" class="IntGraph (strict)"("Y Scale.Range:Maximum"=w866) -> ()  [unwired: 2 in, 2 out]
          }
          event "Image1": Mouse Up {
            n503 = event-data() -> ("Coords"=w887:T11)  [unwired: 1 in, 3 out]
            n504 = stacked-sequence {
              tunnel: w887 -> [w908 _]
              tunnel: w886 -> [_ _]
              tunnel: w885 -> [_ w910]
              tunnel: w884 -> [_ w909]
              frame #0 {
                # "Useless code.  Get rid of if keeping reading of coordinates  by cursor."
                n505 = Unbundle By Name(w908) -> ("Horizontal"=w893:i32, "Vertical"=w889:i32)
                n506 = property on="Image1" class="IntGraph (strict)"() -> ("Y Scale.Range:Maximum"=w900:dbl)  [unwired: 2 in, 2 out]
                n507 = Subtract(x=w893, y=135.0) -> (x-y=w892:dbl)
                n508 = property on="Image1" class="IntGraph (strict)"() -> ("Y Scale.Range:Minimum"=w901:dbl)  [unwired: 2 in, 2 out]
                n509 = property on="Image1" class="IntGraph (strict)"() -> ("X Scale.Range:Minimum"=w902:dbl)  [unwired: 2 in, 2 out]
                n510 = property on="Image1" class="IntGraph (strict)"() -> ("X Scale.Range:Maximum"=w903:dbl)  [unwired: 2 in, 2 out]
                n511 = Subtract(x=w889, y=105) -> (x-y=w904:i32)
                n512 = Divide(x=w904, y=456) -> (x/y=w905:dbl)
                n513 = Divide(x=w892, y=257.0) -> (x/y=w907:dbl)
                n514 = Subtract(x=w903, y=w902) -> (x-y=w896:dbl)
                n515 = Subtract(x=w900, y=w901) -> (x-y=w895:dbl)
                n516 = Multiply(x=w907, y=w896) -> (x*y=w906:dbl)
                n517 = Multiply(x=w905, y=w895) -> (x*y=w899:dbl)
                n518 = Add(x=w906, y=w902) -> (x+y=w898:dbl)
                n519 = Subtract(x=w900, y=w899) -> (x-y=w897:dbl)
                n520 = property on="Image1" class="IntGraph (strict)"("Cursor.Cursor Position:Cursor X"=w898) -> ()  [unwired: 2 in, 2 out]
                n521 = property on="Image1" class="IntGraph (strict)"("Cursor.Cursor Position:Cursor Y"=w897) -> ()  [unwired: 2 in, 2 out]
              }
              frame #1 {
                n522 = Enqueue Element(queue=w909, element=T8 {"Command"="UPDATE_ZOOM", "Parameter"=""}, error in (no error)=w910) -> ()  [unwired: 1 in, 3 out]
              }
            }
          }
          event "Image2": Mouse Up {
            n523 = event-data() -> ("Coords"=w912:T11)  [unwired: 1 in, 7 out]
            n524 = stacked-sequence {
              tunnel: w914 -> [_ w937]
              tunnel: w913 -> [_ w936]
              tunnel: w912 -> [w921 _]
              frame #0 {
                n525 = Unbundle By Name(w921) -> ("Horizontal"=w927:i32, "Vertical"=w923:i32)
                n526 = property on="Image2" class="IntGraph (strict)"() -> ("Y Scale.Range:Maximum"=w917:dbl)  [unwired: 2 in, 2 out]
                n527 = property on="Image2" class="IntGraph (strict)"() -> ("Y Scale.Range:Minimum"=w916:dbl)  [unwired: 2 in, 2 out]
                n528 = property on="Image2" class="IntGraph (strict)"() -> ("X Scale.Range:Maximum"=w920:dbl)  [unwired: 2 in, 2 out]
                n529 = property on="Image2" class="IntGraph (strict)"() -> ("X Scale.Range:Minimum"=w919:dbl)  [unwired: 2 in, 2 out]
                n530 = Subtract(x=w927, y=135.0) -> (x-y=w926:dbl)
                n531 = Subtract(x=w923, y=105) -> (x-y=w932:i32)
                n532 = Divide(x=w932, y=456) -> (x/y=w933:dbl)
                n533 = Divide(x=w926, y=257.0) -> (x/y=w935:dbl)
                n534 = Subtract(x=w920, y=w919) -> (x-y=w930:dbl)
                n535 = Subtract(x=w917, y=w916) -> (x-y=w929:dbl)
                n536 = Multiply(x=w935, y=w930) -> (x*y=w934:dbl)
                n537 = Multiply(x=w933, y=w929) -> (x*y=w931:dbl)
                n538 = Add(x=w934, y=w919) -> (x+y=w918:dbl)
                n539 = Subtract(x=w917, y=w931) -> (x-y=w915:dbl)
                n540 = property on="Image2" class="IntGraph (strict)"("Cursor.Cursor Position:Cursor X"=w918) -> ()  [unwired: 2 in, 2 out]
                n541 = property on="Image2" class="IntGraph (strict)"("Cursor.Cursor Position:Cursor Y"=w915) -> ()  [unwired: 2 in, 2 out]
              }
              frame #1 {
                n542 = Enqueue Element(queue=w937, element=T8 {"Command"="UPDATE_ZOOM", "Parameter"=""}, error in (no error)=w936) -> ()  [unwired: 1 in, 3 out]
              }
            }
          }
          event "LoadSlit": Mouse Up {
            n543 = event-data() -> ()  [unwired: 1 in, 8 out]
            n544 = local read "X 2"() -> (w942:dbl)
            n545 = local read "Y 2"() -> (w941:dbl)
            n546 = local read "Slit Positions"() -> (w943:T5)
            n547 = case shown="0, Default" "SlitSelection" {
              tunnel: [w948 w951 w955] -> w940
              tunnel: w943 -> [w947 w952 w956]
              tunnel: w942 -> [w946 w950 w954]
              tunnel: w941 -> [w945 w949 w953]
              frame 0, Default {
                n548 = Bundle By Name(cluster=w947, "Slit x1"=w946, "Slit y1"=w945) -> (w948:T5)
              }
              frame 1 {
                n549 = Bundle By Name(cluster=w952, "Slit x2"=w950, "Slit y2"=w949) -> (w951:T5)
              }
              frame 2 {
                n550 = Bundle By Name(cluster=w956, "Slit x3"=w954, "Slit y3"=w953) -> (w955:T5)
              }
            }
            n551 = local write "Status 2"("Coordinates Sent to Calculator" ("Status")) -> ()
            n552 = local write "Slit Positions"(w940) -> ()
          }
          event "LoadStar": Mouse Up {
            n553 = event-data() -> ()  [unwired: 1 in, 8 out]
            n554 = local read "X"() -> (w961:dbl)
            n555 = local read "Y"() -> (w960:dbl)
            n556 = local read "Star Positions"() -> (w962:T6)
            n557 = case shown="1" "StarSelection" {
              tunnel: [w966 w969 w973] -> w958
              tunnel: w962 -> [w965 w970 w974]
              tunnel: w961 -> [w964 w968 w972]
              tunnel: w960 -> [w963 w967 w971]
              frame 0, Default {
                n558 = Bundle By Name(cluster=w965, "Star x1"=w964, "Star y1"=w963) -> (w966:T6)
              }
              frame 1 {
                n559 = Bundle By Name(cluster=w970, "Star x2"=w968, "Star y2"=w967) -> (w969:T6)
              }
              frame 2 {
                n560 = Bundle By Name(cluster=w974, "Star x3"=w972, "Star y3"=w971) -> (w973:T6)
              }
            }
            n561 = local write "Status 1"("Coordinates Sent to Calculator" ("Status")) -> ()
            n562 = local write "Star Positions"(w958) -> ()
          }
          event "Image Scale Stretch": Mouse Up {
            n563 = event-data() -> ()  [unwired: 1 in, 9 out]
            n564 = Enqueue Element(queue=w976, element=T8 {"Command"="SCALE_IMAGE", "Parameter"=""}, error in (no error)=w975) -> ()  [unwired: 1 in, 3 out]
          }
          event "Image Scale Stretch 2": Mouse Up {
            n565 = event-data() -> ()  [unwired: 1 in, 8 out]
            n566 = Enqueue Element(queue=w979, element=T8 {"Command"="SCALE_IMAGE", "Parameter"=""}, error in (no error)=w978) -> ()  [unwired: 1 in, 3 out]
          }
          event "Calculate Shifts": Mouse Up {
            # "These are for if you want to display the new coordinates on the GUI. It is currently disabled. To change, right click then select Show Indicator."
            n567 = event-data() -> ()  [unwired: 1 in, 8 out]
            n568 = call "MultislitCalc.vi"("Slit Positions"="Slit Positions", "Star Positions"="Star Positions") -> ("test2"=→"new y1":dbl, "test1"=→"new x1":dbl, "Shifts"=→"Offsets and Rotation":T7)  [unwired: 3 in]
          }
          event "Set Values to Zero": Value Change {
            n569 = event-data() -> ()  [unwired: 1 in, 6 out]
            n570 = Bundle("Delta Theta"=0.0, "Delta X"=0.0, "Delta Y"=0.0, "Delta Theta"=0.0, "Delta X"=0.0, "Delta Y"=0.0) -> (w996:T12)  [unwired: 1 in]
            n571 = Bundle("Delta Theta"=0.0, "Delta X"=0.0, "Delta Y"=0.0) -> (w1000:T7)  [unwired: 1 in]
            n572 = Bundle("Delta Theta"=0.0, "Delta X"=0.0, "Delta Y"=0.0, "Delta Theta"=0.0, "Delta X"=0.0, "Delta Y"=0.0) -> (w986:T12)  [unwired: 1 in]
            n573 = local write "Offsets and Rotation"(w1000) -> ()
            n574 = local write "Star Positions"(w996) -> ()
            n575 = local write "Slit Positions"(w986) -> ()
          }
        }
      }
      frame "SHUTDOWN" {
        n576 = Flush Queue(queue=w1012, error in (no error)=w1011) -> (queue out=w1010:refnum<queue>, error out=w1009:errorcluster)  [unwired: 1 out]
        n577 = Release Queue(queue=w1010, error in (no error)=w1009) -> ()  [unwired: 1 in, 3 out]
        n578 = Current VI's Path() -> (path=w1007:path)
        n579 = Strip Path(path=w1007) -> (name=w1006:string)  [unwired: 1 out]
        n580 = String To Path(string=w1006) -> (path=w1005:path)
        n581 = Open VI Reference(vi path=w1005) -> (vi reference=w1008:refnum<vi>)  [unwired: 5 in, 1 out]
        n582 = invoke class="VI" method="FP.Close"(reference=w1008) -> (reference out=w1004:refnum<vi>)  [unwired: 2 in, 2 out]
        n583 = Close Reference(reference=w1004) -> ()  [unwired: 1 in, 1 out]
      }
      frame "FIT_GAUSSIAN" {
        n584 = case shown="\"Stars\", Default" w1013 {
          tunnel: [w1028 w1029] -> w1014
          frame "Stars", Default {
            n585 = local read "Gauss Fit Window"() -> (w1028:i16[][])
          }
          frame "Slits" {
            n586 = local read "Gauss Fit Window 2"() -> (w1029:i16[][])
          }
        }
        n587 = Multiply(x=w1016, y=0.15) -> (x*y=w1020:T2)
        n588 = Array Size(array=w1014) -> (size(s)=w1024:i32[])
        n589 = Unbundle By Name(w1020) -> ("Serial Binning"=w1022:dbl, "Parallel Binning"=w1021:dbl)
        n590 = Index Array(array=w1024, index=1) -> (element=w1023:i32)
        n591 = Index Array(array=w1024, index=0) -> (element=w1026:i32)
        n592 = stacked-sequence {
          seq-local: [w1030 _ _ _ _ _] -> [_ _ w1067 _ _ w1107]
          seq-local: [_ w1043 _ _ _ _] -> [_ _ w1068 _ w1101 _]
          seq-local: [_ _ w1063 _ _ _] -> [_ _ _ w1097 _ _]
          tunnel: w1014 -> [w1036 w1047 _ _ w1106 w1110]
          tunnel: w1026 -> [w1033 w1046 _ _ _ _]
          tunnel: w1023 -> [w1032 w1045 _ _ _ _]
          tunnel: w1018 -> [_ _ _ w1094 _ _]
          tunnel: w1017 -> [_ _ _ w1095 _ _]
          tunnel: [_ _ _ _ w1103 _] -> _
          tunnel: [_ _ _ _ _ w1108] -> _
          tunnel: w1022 -> [_ _ _ _ w1104 _]
          tunnel: w1021 -> [_ _ _ _ _ w1109]
          tunnel: w1013 -> [_ _ w1062 w1089 _ _]
          frame #0 {
            n593 = Initialize Array(0 ("element"), w1032) -> (w1035:i32[])
            n594 = for {
              N: w1033 -> [_]
              tunnel: w1036 -> [w1042]
              shift-right: [w1041] -> w1031
              shift-left: w1035 -> [w1039]
              i -> [w1037]
              n595 = Index Array(array=w1042, index (row)=w1037) -> (element=w1040:i16[])  [unwired: 1 in]
              n596 = Add(x=w1040, y=w1039) -> (x+y=w1038:i32[])
              n597 = Replace Array Subset(array=w1039, new element=w1038) -> (w1041:i32[])  [unwired: 1 in]
            }
            n598 = call "Fit_1D_Gaussian.vi"("Input 1D Array"=w1031) -> ("center"=w1030:dbl)  [unwired: 3 in, 1 out]
          }
          frame #1 {
            n599 = Initialize Array(0 ("element"), w1046) -> (w1049:i32[])
            n600 = for {
              N: w1045 -> [_]
              tunnel: w1047 -> [w1055]
              shift-right: [w1054] -> w1044
              shift-left: w1049 -> [w1051]
              i -> [w1050]
              n601 = Index Array(array=w1055, index (col)=w1050) -> (element=w1052:i16[])  [unwired: 1 in]
              n602 = Add(x=w1052, y=w1051) -> (x+y=w1053:i32[])
              n603 = Replace Array Subset(array=w1051, new element=w1053) -> (w1054:i32[])  [unwired: 1 in]
            }
            n604 = call "Fit_1D_Gaussian.vi"("Input 1D Array"=w1044) -> ("center"=w1043:dbl)  [unwired: 3 in, 1 out]
          }
          frame #2 {
            # "seemed to be a -2 pixel offset in y for the mask fit"
            n605 = case shown="\"Slits\"" w1062 {
              tunnel: [w1079 w1087] -> w1061
              tunnel: [w1078 w1080] -> w1056
              tunnel: [w1077 w1083] -> w1060
              tunnel: [w1076 w1084] -> w1059
              tunnel: [w1075 w1085] -> w1058
              tunnel: [w1074 w1086] -> w1057
              frame "Stars", Default {
                n606 = property on="Zoom Window" class="IntGraph (strict)"() -> ("X Scale.Range:Minimum"=w1075:dbl)  [unwired: 2 in, 2 out]
                n607 = property on="Zoom Window" class="IntGraph (strict)"() -> ("Y Scale.Range:Minimum"=w1077:dbl)  [unwired: 2 in, 2 out]
                n608 = property on="Zoom Window" class="IntGraph (strict)"() -> ("X Scale.Range:Maximum"=w1074:dbl)  [unwired: 2 in, 2 out]
                n609 = property on="Zoom Window" class="IntGraph (strict)"() -> ("Y Scale.Range:Maximum"=w1076:dbl)  [unwired: 2 in, 2 out]
                n610 = local read "X"() -> (w1079:dbl)
                n611 = local read "Y"() -> (w1078:dbl)
              }
              frame "Slits" {
                n612 = property on="Zoom Window 2" class="IntGraph (strict)"() -> ("X Scale.Range:Maximum"=w1086:dbl)  [unwired: 2 in, 2 out]
                n613 = property on="Zoom Window 2" class="IntGraph (strict)"() -> ("X Scale.Range:Minimum"=w1085:dbl)  [unwired: 2 in, 2 out]
                n614 = property on="Zoom Window 2" class="IntGraph (strict)"() -> ("Y Scale.Range:Maximum"=w1084:dbl)  [unwired: 2 in, 2 out]
                n615 = property on="Zoom Window 2" class="IntGraph (strict)"() -> ("Y Scale.Range:Minimum"=w1083:dbl)  [unwired: 2 in, 2 out]
                n616 = local read "Y 2"() -> (w1081:dbl)
                n617 = local read "X 2"() -> (w1087:dbl)
                n618 = Add(x=w1081, y=2) -> (x+y=w1080:dbl)
              }
            }
            n619 = Subtract(x=w1059, y=w1060) -> (x-y=w1066:dbl)
            n620 = Subtract(x=w1057, y=w1058) -> (x-y=w1065:dbl)
            n621 = Bundle("X 2"=w1061, "Y"=w1056) -> (w1071:cluster{"X 2":dbl, "Y":dbl})  [unwired: 1 in]
            n622 = Bundle(w1065, w1066) -> (w1069:cluster{dbl, dbl})  [unwired: 1 in]
            n623 = Bundle("center"=w1068, "center"=w1067) -> (w1072:cluster{"center":dbl, "center":dbl})  [unwired: 1 in]
            n624 = Divide(x=w1069, y=2) -> (x/y=w1064:cluster{dbl, dbl})
            n625 = Subtract(x=w1072, y=w1064) -> (x-y=w1070:cluster{dbl, dbl})
            n626 = Add(x=w1070, y=w1071) -> (x+y=w1063:cluster{dbl, dbl})
          }
          frame #3 {
            n627 = local read "Display Binning"() -> (w1091:i16)
            n628 = Enqueue Element(queue=w1094, element=T8 {"Command"="UPDATE_ZOOM", "Parameter"=""}, error in (no error)=w1095) -> ()  [unwired: 1 in, 3 out]
            n629 = Equal To 0?(x=w1091) -> (x = 0?=w1092:bool)
            n630 = Select(t=u16 1, s=w1092, f=w1091) -> (s? t:f=w1090:u16)
            n631 = To Double Precision Float(number=w1090) -> (double precision float=w1098:dbl)
            n632 = Divide(x=w1097, y=w1098) -> (x/y=w1088:cluster{dbl, dbl})
            n633 = case shown="\"Slits\"" w1089 {
              tunnel: w1088 -> [w1099 w1100]
              frame "Stars", Default {
                n634 = property on="Image1" class="IntGraph (strict)"("Cursor.Cursor Position"=w1099) -> ()  [unwired: 2 in, 2 out]
              }
              frame "Slits" {
                n635 = property on="Image2" class="IntGraph (strict)"("Cursor.Cursor Position"=w1100) -> ()  [unwired: 2 in, 2 out]
              }
            }
          }
          frame #4 {
            n636 = Index Array(array=w1106, index (row)=w1101) -> (element=w1102:i16[])  [unwired: 1 in]
            n637 = call "Fit_1D_Gaussian.vi"("Input 1D Array"=w1102) -> ("FWHM"=w1105:dbl)  [unwired: 3 in, 1 out]
            n638 = Multiply(x=w1105, y=w1104) -> (x*y=w1103:dbl)
          }
          frame #5 {
            n639 = Index Array(array=w1110, index (col)=w1107) -> (element=w1111:i16[])  [unwired: 1 in]
            n640 = call "Fit_1D_Gaussian.vi"("Input 1D Array"=w1111) -> ("FWHM"=w1112:dbl)  [unwired: 3 in, 1 out]
            n641 = Multiply(x=w1112, y=w1109) -> (x*y=w1108:dbl)
          }
        }
        n642 = local write "Status 1"("Centering star..." ("Image Status")) -> ()
      }
      frame "SCALE_IMAGE" {
        n643 = case shown="\"Stars\", Default" w1113 {
          frame "Stars", Default {
            n644 = local read "Image1"() -> (w1116:dbl[][])
            n645 = Unbundle("Image Scale Stretch") -> (w1123:dbl, w1126:dbl)
            n646 = Array Max & Min(array=w1116) -> ()  [unwired: 4 out]
            n647 = Array Size(array=w1116) -> (size(s)=w1117:i32[])
            n648 = Multiply Array Elements(1:w1117) -> (0:w1119:i32)
            n649 = Add Array Elements(numeric array=w1116) -> (sum=w1118:dbl)
            n650 = Divide(x=w1118, y=w1119) -> (x/y=w1129:dbl)
            n651 = property on="Zoom Window" class="IntGraph (strict)"("Z Scale.Mapping Mode"=u8 1) -> ()  [unwired: 2 in, 2 out]
            n652 = Divide(x=w1126, y=50.0) -> (x/y=w1125:dbl)
            n653 = Multiply(x=w1125, y=w1129) -> (x*y=w1128:dbl)
            n654 = Divide(x=w1123, y=90.0) -> (x/y=w1115:dbl)
            n655 = Multiply(x=w1115, y=w1129) -> (x*y=w1127:dbl)
            n656 = property on="Image1" class="IntGraph (strict)"("Z Scale.Range:Maximum"=w1128) -> ()  [unwired: 2 in, 2 out]
            n657 = property on="Zoom Window" class="IntGraph (strict)"("Z Scale.Range:Maximum"=w1128) -> ()  [unwired: 2 in, 2 out]
            n658 = property on="Zoom Window" class="IntGraph (strict)"("Z Scale.Range:Minimum"=w1127) -> ()  [unwired: 2 in, 2 out]
            n659 = property on="Image1" class="IntGraph (strict)"("Z Scale.Range:Minimum"=w1127) -> ()  [unwired: 2 in, 2 out]
            n660 = local write "Status 1"("Scaling image..." ("Status")) -> ()
          }
          frame "Slits" {
            n661 = local read "Image2"() -> (w1134:dbl[][])
            n662 = Unbundle("Image Scale Stretch 2") -> (w1141:dbl, w1144:dbl)
            n663 = Array Max & Min(array=w1134) -> ()  [unwired: 4 out]
            n664 = Array Size(array=w1134) -> (size(s)=w1138:i32[])
            n665 = Multiply Array Elements(1:w1138) -> (0:w1140:i32)
            n666 = property on="Zoom Window 2" class="IntGraph (strict)"("Z Scale.Mapping Mode"=1) -> ()  [unwired: 2 in, 2 out]
            n667 = Add Array Elements(numeric array=w1134) -> (sum=w1139:dbl)
            n668 = Divide(x=w1139, y=w1140) -> (x/y=w1145:dbl)
            n669 = Divide(x=w1144, y=50.0) -> (x/y=w1143:dbl)
            n670 = Multiply(x=w1143, y=w1145) -> (x*y=w1132:dbl)
            n671 = Divide(x=w1141, y=90.0) -> (x/y=w1137:dbl)
            n672 = Multiply(x=w1137, y=w1145) -> (x*y=w1133:dbl)
            n673 = local write "Status 2"("Scaling image..." ("Status")) -> ()
            n674 = property on="Image2" class="IntGraph (strict)"("Z Scale.Range:Minimum"=w1133) -> ()  [unwired: 2 in, 2 out]
            n675 = property on="Zoom Window 2" class="IntGraph (strict)"("Z Scale.Range:Minimum"=w1133) -> ()  [unwired: 2 in, 2 out]
            n676 = property on="Image2" class="IntGraph (strict)"("Z Scale.Range:Maximum"=w1132) -> ()  [unwired: 2 in, 2 out]
            n677 = property on="Zoom Window 2" class="IntGraph (strict)"("Z Scale.Range:Maximum"=w1132) -> ()  [unwired: 2 in, 2 out]
          }
        }
      }
      frame "UPDATE_ZOOM" {
        n678 = case shown="\"Slits\"" w1148 {
          tunnel: w1147 -> [w1149 _]
          tunnel: w1146 -> [_ w1183]
          frame "Stars", Default {
            n679 = local read "Display Binning"() -> (w1179:i16)
            n680 = property on="Image1" class="IntGraph (strict)"() -> ("Cursor.Cursor Position"=w1152:T13)  [unwired: 2 in, 2 out]
            n681 = Equal To 0?(x=w1179) -> (x = 0?=w1177:bool)
            n682 = Select(t=u16 1, s=w1177, f=w1179) -> (s? t:f=w1178:u16)
            n683 = Multiply(x=w1152, y=w1178) -> (x*y=w1153:T13)
            n684 = Unbundle(w1153) -> ("Cursor X"=w1173:dbl, "Cursor Y"=w1172:dbl)
            n685 = property on="Image1" class="IntGraph (strict)"() -> ("Bounds:Area Width"=w1157:u32)  [unwired: 2 in, 2 out]
            n686 = Index Array(array=w1149, index (row)=w1173, index (col)=w1172) -> (element=→"Value":i16)
            n687 = Increment(x=w1173) -> (x+1=→"X":dbl)
            n688 = Increment(x=w1172) -> (x+1=→"Y":dbl)
            n689 = Divide(x=w1157, y="Zoom Window Width (1/x)") -> (x/y=w1158:dbl)
            n690 = property on="Image1" class="IntGraph (strict)"() -> ("Bounds:Area Height"=w1162:u32)  [unwired: 2 in, 2 out]
            n691 = To Word Integer(number=w1158) -> (16bit integer=w1163:i16)
            n692 = Divide(x=w1163, y=2.0) -> (x/y=w1155:dbl)
            n693 = Divide(x=w1162, y="Zoom Window Width (1/x)") -> (x/y=w1161:dbl)
            n694 = To Word Integer(number=w1155) -> (16bit integer=w1156:i16)
            n695 = To Word Integer(number=w1161) -> (16bit integer=w1164:i16)
            n696 = Subtract(x=w1173, y=w1156) -> (x-y=w1170:dbl)
            n697 = Divide(x=w1164, y=2.0) -> (x/y=w1160:dbl)
            n698 = To Word Integer(number=w1160) -> (16bit integer=w1165:i16)
            n699 = Subtract(x=w1172, y=w1165) -> (x-y=w1168:dbl)
            n700 = To Word Integer(number=w1170) -> (16bit integer=w1171:i16)
            n701 = To Word Integer(number=w1168) -> (16bit integer=w1169:i16)
            n702 = Array Subset(array=w1149, index (row)=w1171, length (row)=w1163, index (col)=w1169, length (col)=w1164) -> (→"Zoom Window":i16[][])
            n703 = Bundle(w1156, w1165) -> (w1166:cluster{i16, i16})  [unwired: 1 in]
            n704 = property on="Zoom Window" class="IntGraph (strict)"("Cursor.Cursor Position"=w1166) -> ()  [unwired: 2 in, 2 out]
          }
          frame "Slits" {
            n705 = property on="Image2" class="IntGraph (strict)"() -> ("Cursor.Cursor Position"=w1182:T13)  [unwired: 2 in, 2 out]
            n706 = local read "Display Binning 2"() -> (w1208:i16)
            n707 = Equal To 0?(x=w1208) -> (x = 0?=w1206:bool)
            n708 = Select(t=u16 1, s=w1206, f=w1208) -> (s? t:f=w1207:u16)
            n709 = Multiply(x=w1182, y=w1207) -> (x*y=w1185:T13)
            n710 = property on="Image2" class="IntGraph (strict)"() -> ("Bounds:Area Width"=w1181:u32)  [unwired: 2 in, 2 out]
            n711 = Unbundle(w1185) -> ("Cursor X"=w1202:dbl, "Cursor Y"=w1201:dbl)
            n712 = Index Array(array=w1183, index (row)=w1202, index (col)=w1201) -> (element=→"Value 2":i16)
            n713 = Increment(x=w1201) -> (x+1=→"Y 2":dbl)
            n714 = Increment(x=w1202) -> (x+1=→"X 2":dbl)
            n715 = Divide(x=w1181, y="Zoom Window Width (1/x) 2") -> (x/y=w1189:dbl)
            n716 = property on="Image2" class="IntGraph (strict)"() -> ("Bounds:Area Height"=w1180:u32)  [unwired: 2 in, 2 out]
            n717 = To Word Integer(number=w1189) -> (16bit integer=w1193:i16)
            n718 = Divide(x=w1193, y=2.0) -> (x/y=w1187:dbl)
            n719 = Divide(x=w1180, y="Zoom Window Width (1/x) 2") -> (x/y=w1192:dbl)
            n720 = To Word Integer(number=w1187) -> (16bit integer=w1188:i16)
            n721 = To Word Integer(number=w1192) -> (16bit integer=w1194:i16)
            n722 = Subtract(x=w1202, y=w1188) -> (x-y=w1199:dbl)
            n723 = Divide(x=w1194, y=2.0) -> (x/y=w1191:dbl)
            n724 = To Word Integer(number=w1191) -> (16bit integer=w1195:i16)
            n725 = Subtract(x=w1201, y=w1195) -> (x-y=w1197:dbl)
            n726 = To Word Integer(number=w1199) -> (16bit integer=w1200:i16)
            n727 = To Word Integer(number=w1197) -> (16bit integer=w1198:i16)
            n728 = Array Subset(array=w1183, index (row)=w1200, length (row)=w1193, index (col)=w1198, length (col)=w1194) -> (→"Zoom Window 2":i16[][])
            n729 = Bundle(w1188, w1195) -> (w1210:cluster{i16, i16})  [unwired: 1 in]
            n730 = property on="Zoom Window 2" class="IntGraph (strict)"("Cursor.Cursor Position"=w1210) -> ()  [unwired: 2 in, 2 out]
          }
        }
      }
      frame "ZOOM_FOR_GAUSS_FIT" {
        n731 = case shown="\"Slits\"" w1213 {
          tunnel: w1212 -> [w1214 _]
          tunnel: w1211 -> [_ w1251]
          frame "Stars", Default {
            n732 = local read "Display Binning"() -> (w1241:i16)
            n733 = property on="Image1" class="IntGraph (strict)"() -> ("Cursor.Cursor Position"=w1235:T13)  [unwired: 2 in, 2 out]
            n734 = local read "Zoom Window Width (1/x)"() -> (w1222:u32)
            n735 = Equal To 0?(x=w1241) -> (x = 0?=w1239:bool)
            n736 = Select(t=u16 1, s=w1239, f=w1241) -> (s? t:f=w1240:u16)
            n737 = property on="Image1" class="IntGraph (strict)"() -> ("Bounds:Area Width"=w1223:u32)  [unwired: 2 in, 2 out]
            n738 = Multiply(x=w1235, y=w1240) -> (x*y=w1234:T13)
            n739 = Unbundle(w1234) -> ("Cursor X"=w1236:dbl, "Cursor Y"=w1237:dbl)
            n740 = Divide(x=w1223, y=w1222) -> (x/y=w1216:dbl)
            n741 = To Word Integer(number=w1216) -> (16bit integer=w1219:i16)
            n742 = property on="Image1" class="IntGraph (strict)"() -> ("Bounds:Area Height"=w1224:u32)  [unwired: 2 in, 2 out]
            n743 = local write "X"(w1236) -> ()
            n744 = Divide(x=w1219, y=2.0) -> (x/y=w1230:dbl)
            n745 = local write "Y"(w1237) -> ()
            n746 = Divide(x=w1224, y=w1222) -> (x/y=w1218:dbl)
            n747 = To Word Integer(number=w1230) -> (16bit integer=w1232:i16)
            n748 = To Word Integer(number=w1218) -> (16bit integer=w1220:i16)
            n749 = Subtract(x=w1236, y=w1232) -> (x-y=w1226:dbl)
            n750 = Divide(x=w1220, y=2.0) -> (x/y=w1231:dbl)
            n751 = To Word Integer(number=w1226) -> (16bit integer=w1227:i16)
            n752 = To Word Integer(number=w1231) -> (16bit integer=w1233:i16)
            n753 = Subtract(x=w1237, y=w1233) -> (x-y=w1229:dbl)
            n754 = To Word Integer(number=w1229) -> (16bit integer=w1228:i16)
            n755 = Array Subset(array=w1214, index (row)=w1227, length (row)=w1219, index (col)=w1228, length (col)=w1220) -> (→"Gauss Fit Window":i16[][])
            n756 = Bundle(w1232, w1233) -> (w1225:cluster{i16, i16})  [unwired: 1 in]
            n757 = property on="Zoom Window" class="IntGraph (strict)"("Cursor.Cursor Position"=w1225) -> ()  [unwired: 2 in, 2 out]
          }
          frame "Slits" {
            n758 = property on="Image2" class="IntGraph (strict)"() -> ("Cursor.Cursor Position"=w1248:T13)  [unwired: 2 in, 2 out]
            n759 = local read "Display Binning 2"() -> (w1246:i16)
            n760 = local read "Zoom Window Width (1/x)"() -> (w1247:u32)
            n761 = Equal To 0?(x=w1246) -> (x = 0?=w1253:bool)
            n762 = property on="Image2" class="IntGraph (strict)"() -> ("Plot Area:Size:Width"=w1250:u32)  [unwired: 2 in, 2 out]
            n763 = Select(t=u16 1, s=w1253, f=w1246) -> (s? t:f=w1252:u16)
            n764 = Multiply(x=w1248, y=w1252) -> (x*y=w1255:T13)
            n765 = Unbundle(w1255) -> ("Cursor X"=w1243:dbl, "Cursor Y"=w1242:dbl)
            n766 = Divide(x=w1250, y=w1247) -> (x/y=w1268:dbl)
            n767 = To Word Integer(number=w1268) -> (16bit integer=w1265:i16)
            n768 = property on="Image2" class="IntGraph (strict)"() -> ("Plot Area:Size:Height"=w1249:u32)  [unwired: 2 in, 2 out]
            n769 = local write "X 2"(w1243) -> ()
            n770 = Divide(x=w1265, y=2.0) -> (x/y=w1259:dbl)
            n771 = Divide(x=w1249, y=w1247) -> (x/y=w1266:dbl)
            n772 = To Word Integer(number=w1259) -> (16bit integer=w1257:i16)
            n773 = local write "Y 2"(w1242) -> ()
            n774 = To Word Integer(number=w1266) -> (16bit integer=w1264:i16)
            n775 = Subtract(x=w1243, y=w1257) -> (x-y=w1263:dbl)
            n776 = Divide(x=w1264, y=2.0) -> (x/y=w1258:dbl)
            n777 = To Word Integer(number=w1263) -> (16bit integer=w1262:i16)
            n778 = To Word Integer(number=w1258) -> (16bit integer=w1256:i16)
            n779 = Subtract(x=w1242, y=w1256) -> (x-y=w1260:dbl)
            n780 = To Word Integer(number=w1260) -> (16bit integer=w1261:i16)
            n781 = Array Subset(array=w1251, index (row)=w1262, length (row)=w1265, index (col)=w1261, length (col)=w1264) -> (→"Gauss Fit Window 2":i16[][])
            n782 = Bundle(w1257, w1256) -> (w1245:cluster{i16, i16})  [unwired: 1 in]
            n783 = property on="Zoom Window 2" class="IntGraph (strict)"("Cursor.Cursor Position"=w1245) -> ()  [unwired: 2 in, 2 out]
          }
        }
      }
      frame "OPEN_FITS_FILE" {
        n784 = String To Path(string=w1274) -> (path=w1275:path)
        n785 = Strip Path(path=w1275) -> (stripped path=w1276:path)  [unwired: 1 out]
        n786 = Path To String(path=w1276) -> (string=w1277:string)
        n787 = Equal?(x=w1277, y=".") -> (x = y?=w1272:bool)
        n788 = case shown="True" w1272 {
          tunnel: [w1283 w1285] -> w1273
          tunnel: w1274 -> [w1283 w1284]
          frame False {
          }
          frame True {
            n789 = Concatenate Strings("C:\\DATA\\", w1284) -> (w1285:string)
          }
        }
        n790 = Not(x=w1272) -> (.not. x?=w1270:bool)
        n791 = Wait (ms)(milliseconds to wait=u32 1000) -> (millisecond timer value=w1279:u32)
        n792 = case shown="True" w1270 {
          tunnel: w1282 -> [_ w1295]
          tunnel: w1281 -> [_ w1292]
          tunnel: w1274 -> [_ w1289]
          tunnel: w1279 -> [_ _]
          tunnel: w1273 -> [_ w1288]
          tunnel: w1271 -> [_ w1287]
          frame False {
          }
          frame True {
            n793 = String To Path(string=w1288) -> (path=w1291:path)
            "Path to Current File" <- w1291
            n794 = call "gfitsio-open-file.vi"("error in (no error)"=w1295, "read only? (T:no)"=TRUE, "path"=w1291) -> ("error out"=w1293:errorcluster, "gfits refnum"=→"gfits refnum":T3)  [unwired: 7 in]
            n795 = case shown="No Error" w1293 {
              selector: w1293 -> [w1310 w1315]
              tunnel: w1292 -> [w1309 _]
              tunnel: w1289 -> [w1298 _]
              tunnel: w1287 -> [w1296 _]
              frame No Error {
                n796 = String To Path(string=w1298) -> (path=w1299:path)
                n797 = Enqueue Element(queue=w1309, element=T8 {"Command"="READ_FITS_HEADER", "Parameter"=""}, error in (no error)=w1310) -> (queue out=w1305:refnum<queue>, error out=w1306:errorcluster)  [unwired: 1 in, 1 out]
                n798 = Strip Path(path=w1299) -> (name=w1297:string)  [unwired: 1 out]
                n799 = case shown="\"Slits\"" w1296 {
                  tunnel: w1297 -> [w1312 w1313]
                  frame "Stars", Default {
                    n800 = property on="Image1" class="IntGraph (strict)"("Caption.Text"=w1312) -> ()  [unwired: 2 in, 2 out]
                  }
                  frame "Slits" {
                    n801 = property on="Image2" class="IntGraph (strict)"("Caption.Text"=w1313) -> ()  [unwired: 2 in, 2 out]
                  }
                }
                n802 = Enqueue Element(queue=w1305, element=T8 {"Command"="CONVERT_FITS_FILE", "Parameter"=""}, error in (no error)=w1306) -> (queue out=w1303:refnum<queue>, error out=w1300:errorcluster)  [unwired: 1 in, 1 out]
                n803 = Enqueue Element(queue=w1303, element=T8 {"Command"="REPAIR_LOST_ROWS", "Parameter"=""}, error in (no error)=w1300) -> (queue out=w1302:refnum<queue>, error out=w1301:errorcluster)  [unwired: 1 in, 1 out]
                n804 = Enqueue Element(queue=w1302, element=T8 {"Command"="DISPLAY_IMAGE", "Parameter"=""}, error in (no error)=w1301) -> ()  [unwired: 1 in, 3 out]
              }
              frame Error {
                n805 = One Button Dialog(message="ERROR:  File could not be found, or access to the FITS file could not be obtained.  ") -> ()  [unwired: 1 in, 1 out]
                "error IO" <- w1315
              }
            }
          }
        }
      }
      frame "READ_FITS_HEADER" {
        n806 = call "gfitsio-get-image-size.vi"("error in (no error)"=w1325, "gfits refnum"=w1326) -> ("naxes"=w1329:i32[], "dup gfits refnum"=w1324:T3)  [unwired: 6 in, 2 out]
        n807 = case shown="\"Blue\", Default" w1316 {
          tunnel: [string[] ["CAM_ANG", "PG5_6", "PG5_11", "GRT_ANG", "PG5_9", "PG5_4", "MOUNT_AZ", "PG5_5", "PG5_10", "POSANGLE", "GRATING"] string[] ["CAM_ANG", "PG3_4", "PG3_0", "GRT_ANG", "PG3_2", "PG3_6", "MOUNT_AZ", "PG3_5", "PG3_1", "POSANGLE", "GRATING"]] -> w1322
          frame "Red" {
            # "(PG3_0=Serial Origin\nPG3_4  =Parallel Origin\nPG3_2 =Serial Binning\nPG3_6= Parallel Binning\nPG3_5 = parallel length\nPG3_1 = serial length"
          }
          frame "Blue", Default {
            # "(PG3_0=Serial Origin\nPG3_4  =Parallel Origin\nPG3_2 =Serial Binning\nPG3_6= Parallel Binning\nPG3_5 = parallel length\nPG3_1 = serial length"
          }
        }
        n808 = Index Array(array=w1329, index=0) -> (element=w1328:i32)
        n809 = Index Array(array=w1329, index=1) -> (element=w1327:i32)
        n810 = Bundle By Name(cluster=w1323, "# Rows (raw)"=w1328, "# Columns (raw)"=w1327) -> (w1320:T2)
        n811 = call "gfitsio-read-header.vi"("gfits refnum"=w1324) -> ("header"=w1319:string[])  [unwired: 8 in, 2 out]
        n812 = for {
          tunnel: w1322 -> [w1345]
          tunnel: w1319 -> [w1338] mode=indexing
          shift-right: [w1343] -> w1321
          shift-left: w1320 -> [w1344]
          shift-right: [w1342] -> _
          shift-left: "" -> [w1336]
          shift-right: [w1335] -> _
          shift-left: "" -> [w1337]
          tunnel: w1316 -> [w1334]
          i -> [w1340]
          n813 = for {
            tunnel: w1338 -> [w1359]
            tunnel: w1345 -> [w1361] mode=indexing
            shift-right: [w1358] -> w1343
            shift-left: w1344 -> [w1357]
            tunnel: w1334 -> [w1356]
            n814 = Match Pattern(string=w1359, regular expression=w1361) -> (after substring=w1360:string, offset past match=w1362:i32)  [unwired: 1 in, 2 out]
            n815 = Less Than 0?(x=w1362) -> (x < 0?=w1363:bool)
            n816 = case shown="False" w1363 {
              tunnel: w1361 -> [w1372 _]
              tunnel: w1357 -> [w1371 w1472]
              tunnel: w1360 -> [w1368 _]
              tunnel: [w1370 w1472] -> w1358
              tunnel: w1356 -> [w1364 _]
              frame False {
                n817 = call <vilib>:"Space Constant.vi"() -> ("String"=w1366:string)
                n818 = String Subset(string=w1368, length (rest)=1) -> (substring=w1367:string)  [unwired: 1 in]
                n819 = Equal?(x=w1366, y=w1367) -> (x = y?=w1365:bool)
                n820 = case shown="True" w1365 {
                  tunnel: w1372 -> [_ w1383]
                  tunnel: w1371 -> [w1373 w1382]
                  tunnel: w1368 -> [_ w1379]
                  tunnel: [w1373 w1377] -> w1370
                  tunnel: w1364 -> [_ w1374]
                  frame False {
                  }
                  frame True {
                    n821 = Match Pattern(string=w1379, regular expression="=") -> (after substring=w1375:string)  [unwired: 1 in, 3 out]
                    n822 = Match Pattern(string=w1375, regular expression="/") -> (before substring=w1376:string)  [unwired: 1 in, 3 out]
                    n823 = Fract/Exp String To Number(string=w1376) -> (number=w1378:dbl)  [unwired: 3 in, 1 out]
                    n824 = case shown="\"Blue\", Default" w1374 {
                      tunnel: w1383 -> [w1388 w1432]
                      tunnel: w1382 -> [w1387 w1431]
                      tunnel: w1378 -> [w1386 w1430]
                      tunnel: [w1384 w1429] -> w1377
                      tunnel: w1375 -> [w1385 w1428]
                      frame "Red" {
                        n825 = case shown="\"PG5_4\"" w1388 {
                          tunnel: w1387 -> [w1389 w1391 w1394 w1397 w1400 w1404 w1405 w1413 w1416 w1420 w1424 w1426]
                          tunnel: w1386 -> [_ w1390 w1393 w1396 w1399 w1403 w1406 _ w1417 w1419 w1422 w1425]
                          tunnel: [w1389 w1392 w1395 w1398 w1401 w1402 w1407 w1412 w1418 w1421 w1423 w1427] -> w1384
                          tunnel: w1385 -> [_ _ _ _ _ _ _ w1414 _ _ _ _]
                          frame "", Default {
                          }
                          frame "PG5_11" {
                            n826 = Bundle By Name(cluster=w1391, "Serial Origin"=w1390) -> (w1392:T2)
                          }
                          frame "PG5_10" {
                            n827 = Bundle By Name(cluster=w1394, "Serial Length"=w1393, "# Columns (raw)"=w1393) -> (w1395:T2)
                          }
                          frame "PG5_9" {
                            n828 = Bundle By Name(cluster=w1397, "Serial Binning"=w1396) -> (w1398:T2)
                          }
                          frame "PG5_6" {
                            n829 = Bundle By Name(cluster=w1400, "Parallel Origin"=w1399) -> (w1401:T2)
                          }
                          frame "PG5_5" {
                            n830 = Bundle By Name(cluster=w1404, "Parallel Length"=w1403, "# Rows (raw)"=w1403) -> (w1402:T2)
                          }
                          frame "POSANGLE" {
                            n831 = Bundle By Name(cluster=w1405, "Pos. Angle"=w1406) -> (w1407:T2)
                          }
                          frame "GRATING" {
                            n832 = Match Pattern(string=w1414, regular expression="_") -> (after substring=w1409:string)  [unwired: 1 in, 3 out]
                            n833 = Match Pattern(string=w1409, regular expression="'") -> (before substring=w1408:string)  [unwired: 1 in, 3 out]
                            n834 = Fract/Exp String To Number(string=w1408) -> (number=w1411:dbl)  [unwired: 3 in, 1 out]
                            n835 = Bundle By Name(cluster=w1413, "Grating"=w1411) -> (w1412:T2)
                          }
                          frame "PG5_4" {
                            n836 = Bundle By Name(cluster=w1416, "Parallel Binning"=w1417) -> (w1418:T2)
                          }
                          frame "CAM_ANG" {
                            n837 = Bundle By Name(cluster=w1420, "Camera Angle"=w1419) -> (w1421:T2)
                          }
                          frame "GRT_ANG" {
                            n838 = Bundle By Name(cluster=w1424, "Grating Angle"=w1422) -> (w1423:T2)
                          }
                          frame "MOUNT_AZ" {
                            n839 = Bundle By Name(cluster=w1426, "Azimuth"=w1425) -> (w1427:T2)
                          }
                        }
                      }
                      frame "Blue", Default {
                        n840 = case shown="\"PG3_6\"" w1432 {
                          tunnel: w1431 -> [w1433 w1435 w1438 w1441 w1444 w1448 w1449 w1457 w1460 w1464 w1468 w1470]
                          tunnel: w1430 -> [_ w1434 w1437 w1440 w1443 w1447 w1450 _ w1461 w1463 w1466 w1469]
                          tunnel: [w1433 w1436 w1439 w1442 w1445 w1446 w1451 w1456 w1462 w1465 w1467 w1471] -> w1429
                          tunnel: w1428 -> [_ _ _ _ _ _ _ w1458 _ _ _ _]
                          frame "", Default {
                          }
                          frame "PG3_0" {
                            n841 = Bundle By Name(cluster=w1435, "Serial Origin"=w1434) -> (w1436:T2)
                          }
                          frame "PG3_1" {
                            n842 = Bundle By Name(cluster=w1438, "Serial Length"=w1437, "# Columns (raw)"=w1437) -> (w1439:T2)
                          }
                          frame "PG3_2" {
                            n843 = Bundle By Name(cluster=w1441, "Serial Binning"=w1440) -> (w1442:T2)
                          }
                          frame "PG3_4" {
                            n844 = Bundle By Name(cluster=w1444, "Parallel Origin"=w1443) -> (w1445:T2)
                          }
                          frame "PG3_5" {
                            n845 = Bundle By Name(cluster=w1448, "Parallel Length"=w1447, "# Rows (raw)"=w1447) -> (w1446:T2)
                          }
                          frame "POSANGLE" {
                            n846 = Bundle By Name(cluster=w1449, "Pos. Angle"=w1450) -> (w1451:T2)
                          }
                          frame "GRATING" {
                            n847 = Match Pattern(string=w1458, regular expression="_") -> (after substring=w1453:string)  [unwired: 1 in, 3 out]
                            n848 = Match Pattern(string=w1453, regular expression="'") -> (before substring=w1452:string)  [unwired: 1 in, 3 out]
                            n849 = Fract/Exp String To Number(string=w1452) -> (number=w1455:dbl)  [unwired: 3 in, 1 out]
                            n850 = Bundle By Name(cluster=w1457, "Grating"=w1455) -> (w1456:T2)
                          }
                          frame "PG3_6" {
                            n851 = Bundle By Name(cluster=w1460, "Parallel Binning"=w1461) -> (w1462:T2)
                          }
                          frame "CAM_ANG" {
                            n852 = Bundle By Name(cluster=w1464, "Camera Angle"=w1463) -> (w1465:T2)
                          }
                          frame "GRT_ANG" {
                            n853 = Bundle By Name(cluster=w1468, "Grating Angle"=w1466) -> (w1467:T2)
                          }
                          frame "MOUNT_AZ" {
                            n854 = Bundle By Name(cluster=w1470, "Azimuth"=w1469) -> (w1471:T2)
                          }
                        }
                      }
                    }
                  }
                }
              }
              frame True {
              }
            }
          }
          n855 = Greater?(x=w1340, y=i8 91) -> (0:w1339:bool)
          n856 = case shown="False" w1339 {
            tunnel: [w1349 ""] -> w1342
            tunnel: w1338 -> [w1348 w1353]
            tunnel: w1337 -> [_ w1354]
            tunnel: w1336 -> [w1347 _]
            tunnel: ["" w1351] -> w1335
            frame False {
              n857 = Concatenate Strings(w1347, w1348, "\r\n") -> (w1349:string)
              "FITS Header" <- w1349
            }
            frame True {
              n858 = Concatenate Strings(w1354, w1353, "\r\n") -> (w1351:string)
              "FITS Header 2" <- w1351
            }
          }
        }
        n859 = local write "Raw Data"(w1321) -> ()
      }
      frame "GET_IMAGE_STATS" {
        n860 = case shown="\"Stars\", Default" w1475 {
          tunnel: w1474 -> [w1479 _]
          tunnel: w1473 -> [_ w1485]
          frame "Stars", Default {
            n861 = Array Size(array=w1479) -> (size(s)=w1481:i32[])
            n862 = Multiply Array Elements(1:w1481) -> (0:w1482:i32)
            n863 = Array Max & Min(array=w1479) -> (max value=w1477:i16, min value=w1476:i16)  [unwired: 2 out]
            n864 = Reshape Array(w1479, w1482) -> (w1483:i16[])
            n865 = To Double Precision Float(number=w1483) -> (double precision float=w1484:dbl[])
            n866 = Add Array Elements(numeric array=w1484) -> (sum=w1480:dbl)
            n867 = Divide(x=w1480, y=w1482) -> (x/y=w1478:dbl)
            n868 = local write "Maximum Pix Value"(w1477) -> ()
            n869 = local write "Minimum Pix Value"(w1476) -> ()
            n870 = local write "Avg Pix Value"(w1478) -> ()
          }
          frame "Slits" {
            n871 = Array Size(array=w1485) -> (size(s)=w1490:i32[])
            n872 = Multiply Array Elements(1:w1490) -> (0:w1491:i32)
            n873 = Array Max & Min(array=w1485) -> (max value=→"Maximum Pix Value":i16, min value=→"Minimum Pix Value":i16)  [unwired: 2 out]
            n874 = Reshape Array(w1485, w1491) -> (w1492:i16[])
            n875 = To Double Precision Float(number=w1492) -> (double precision float=w1493:dbl[])
            n876 = Add Array Elements(numeric array=w1493) -> (sum=w1486:dbl)
            n877 = Divide(x=w1486, y=w1491) -> (x/y=→"Avg Pix Value":dbl)
          }
        }
      }
    }
    n878 = Equal?(x=w23, y="SHUTDOWN") -> (x = y?=w24:bool)
  }
  n879 = property on="Raw Data" class="Clust (strict)"("Visible"=TRUE) -> ()  [unwired: 2 in, 2 out]
